vi "03 cDAQ Chan Tester.vi"(7 "Tasks In":refnum<k21>[](array[refnum]), 8 "error in (no error)":errorcluster, 9 "Stream Voltages to File":bool, 10 "DC Voltages Filename":path, 11 "Mode":T1(ring)) -> (0 "error out":errorcluster, 2 "CDAQ Data Out":dbl[](array[numeric]), 5 "Tasks Out":refnum<k21>[](array[refnum]))   [LabVIEW 2012]
uses:
  Hybrid Water Heater/Experiments/Sensor.ctl
  <vilib>/DAQmx/read.llb/DAQmx Read (Analog 2D DBL NChan NSamp).vi
  <vilib>/DAQmx/miscellaneous.llb/DAQmx Fill In Error Info.vi
  Global Test Variables DPT.vi
  <vilib>/Analysis/NI_AALBase.lvlib
  <resource>/objmgr/daqmx.rc
panel:
  in  "I.DC Event":i32=14
  in  "I.AC Event":i32=6
  out "AC Events":cluster{"Mean":dbl, "StdDev":dbl}[](array[cluster])
  out "DC Voltages":cluster{"Mean":dbl, "StdDev":dbl}[](array[cluster])
  in  "Tab Control":enum32{"Graph", "Settings"}(tab)
  out "Voltages":dbl[][](graph)
  out "AvailSampPerAIChan":u32
  out "AvailSampPerTempChan":u32
  in  "TC Max OK Val":dbl=400.0
  in  "TC Min OK Val":dbl=20.0
  in  "StDev Thresh":dbl=0.2
  in  "Timeout":i32=1000
  out "Temps data":dbl[][](array[numeric]) format="%0.2f"
  out "AI Data":dbl[][](array[numeric]) format="%0.2f"
  out "error ai":errorcluster
  in  "Rate_T":dbl=16.0 caption="Rate" format="%0.2f"
  in  "Rate_AI":dbl=16.0
  in  "CDAQ Data":dbl[](array[numeric])
  in  "End":bool
  in  "I.Bar":i32=5
  out "Bar":cluster{"Mean":dbl, "StdDev":dbl}
  in  "I.Gvol":i32=3
  out "G.Vol":cluster{"Mean":dbl, "StdDev":dbl}
  out "Weight":cluster{"Mean":dbl, "StdDev":dbl}
  in  "I.W":i32=1
  in  "I.Tmp":i32=4
  out "Temp":cluster{"Mean":dbl, "StdDev":dbl}
  out "RH":cluster{"Mean":dbl, "StdDev":dbl}
  in  "I.RH":i32=2
  out "G.Pres.":cluster{"Mean":dbl, "StdDev":dbl}
  in  "I.Gas Pressure":i32
  out "Count":dbl
  in  "Panel 4":T2[][](array[typedef])=[[{"Mean"=0.0, " Std"=0.0, "Color Box"=8585007}, {"Mean"=0.0, " Std"=0.0, "Color Box"=8585007}, {"Mean"=0.0, " Std"=0.0, "Color Box"=8585007}, {"Mean"=0.0, " Std"=0.0, "Color Box"=8585007}, {"Mean"=0.0, " Std"=0.0, "Color Box"=8585007}, {"Mean"=0.0, " Std"=0.0, "Color Box"=8585007}], [{"Mean"=0.0, " Std"=0.0, "Color Box"=8585007}, {"Mean"=0.0, " Std"=0.0, "Color Box"=8585007}, {"Mean"=0.0, " Std"=0.0, "Color Box"=8585007}, {"Mean"=0.0, " Std"=0.0, "Color Box"=8585007}, {"Mean"=0.0, " Std"=0.0, "Color Box"=8585007}, {"Mean"=0.0, " Std"=0.0, "Color Box"=8585007}], [{"Mean"=0.0, " Std"=0.0, "Color Box"=8585007}, {"Mean"=0.0, " Std"=0.0, "Color Box"=8585007}, {"Mean"=0.0, " Std"=0.0, "Color Box"=8585007}, {"Mean"=0.0, " Std"=0.0, "Color Box"=8585007}, {"Mean"=0.0, " Std"=0.0, "Color Box"=8585007}, {"Mean"=0.0, " Std"=0.0, "Color Box"=8585007}]]
  out "Gas Temp":T2={"Mean"=0.0, " Std"=0.0, "Color Box"=8585007}
  in  "Panel 3":T2[][](array[typedef])=[[{"Mean"=0.0, " Std"=0.0, "Color Box"=8585007}, {"Mean"=0.0, " Std"=0.0, "Color Box"=8585007}, {"Mean"=0.0, " Std"=0.0, "Color Box"=8585007}, {"Mean"=0.0, " Std"=0.0, "Color Box"=8585007}, {"Mean"=0.0, " Std"=0.0, "Color Box"=8585007}, {"Mean"=0.0, " Std"=0.0, "Color Box"=8585007}], [{"Mean"=0.0, " Std"=0.0, "Color Box"=8585007}, {"Mean"=0.0, " Std"=0.0, "Color Box"=8585007}, {"Mean"=0.0, " Std"=0.0, "Color Box"=8585007}, {"Mean"=0.0, " Std"=0.0, "Color Box"=8585007}, {"Mean"=0.0, " Std"=0.0, "Color Box"=8585007}, {"Mean"=0.0, " Std"=0.0, "Color Box"=8585007}], [{"Mean"=0.0, " Std"=0.0, "Color Box"=8585007}, {"Mean"=0.0, " Std"=0.0, "Color Box"=8585007}, {"Mean"=0.0, " Std"=0.0, "Color Box"=8585007}, {"Mean"=0.0, " Std"=0.0, "Color Box"=8585007}, {"Mean"=0.0, " Std"=0.0, "Color Box"=8585007}, {"Mean"=0.0, " Std"=0.0, "Color Box"=8585007}]]
  in  "Panel 2":T2[][](array[typedef])=[[{"Mean"=0.0, " Std"=0.0, "Color Box"=8585007}, {"Mean"=0.0, " Std"=0.0, "Color Box"=8585007}, {"Mean"=0.0, " Std"=0.0, "Color Box"=8585007}, {"Mean"=0.0, " Std"=0.0, "Color Box"=8585007}, {"Mean"=0.0, " Std"=0.0, "Color Box"=8585007}, {"Mean"=0.0, " Std"=0.0, "Color Box"=8585007}], [{"Mean"=0.0, " Std"=0.0, "Color Box"=8585007}, {"Mean"=0.0, " Std"=0.0, "Color Box"=8585007}, {"Mean"=0.0, " Std"=0.0, "Color Box"=8585007}, {"Mean"=0.0, " Std"=0.0, "Color Box"=8585007}, {"Mean"=0.0, " Std"=0.0, "Color Box"=8585007}, {"Mean"=0.0, " Std"=0.0, "Color Box"=8585007}], [{"Mean"=0.0, " Std"=0.0, "Color Box"=8585007}, {"Mean"=0.0, " Std"=0.0, "Color Box"=8585007}, {"Mean"=0.0, " Std"=0.0, "Color Box"=8585007}, {"Mean"=0.0, " Std"=0.0, "Color Box"=8585007}, {"Mean"=0.0, " Std"=0.0, "Color Box"=8585007}, {"Mean"=0.0, " Std"=0.0, "Color Box"=8585007}]]
  in  "Panel 1":T2[][](array[typedef])=[[{"Mean"=0.0, " Std"=0.0, "Color Box"=8585007}, {"Mean"=0.0, " Std"=0.0, "Color Box"=8585007}, {"Mean"=0.0, " Std"=0.0, "Color Box"=8585007}, {"Mean"=0.0, " Std"=0.0, "Color Box"=8585007}, {"Mean"=0.0, " Std"=0.0, "Color Box"=8585007}, {"Mean"=0.0, " Std"=0.0, "Color Box"=8585007}], [{"Mean"=0.0, " Std"=0.0, "Color Box"=8585007}, {"Mean"=0.0, " Std"=0.0, "Color Box"=8585007}, {"Mean"=0.0, " Std"=0.0, "Color Box"=8585007}, {"Mean"=0.0, " Std"=0.0, "Color Box"=8585007}, {"Mean"=0.0, " Std"=0.0, "Color Box"=8585007}, {"Mean"=0.0, " Std"=0.0, "Color Box"=8585007}], [{"Mean"=0.0, " Std"=0.0, "Color Box"=8585007}, {"Mean"=0.0, " Std"=0.0, "Color Box"=8585007}, {"Mean"=0.0, " Std"=0.0, "Color Box"=8585007}, {"Mean"=0.0, " Std"=0.0, "Color Box"=8585007}, {"Mean"=0.0, " Std"=0.0, "Color Box"=8585007}, {"Mean"=0.0, " Std"=0.0, "Color Box"=8585007}]]
  in  "Num Samples":i32=5
  in  "Test DAQ":bool
  in  "EXIT":bool
  # "DPT Pannel Channel Tester"
  # "Channel \nGas Pressure 0\nWeight 1\nRH 2\nGas Volume 3\nTemp 4\nBaromentric Pressure 5"
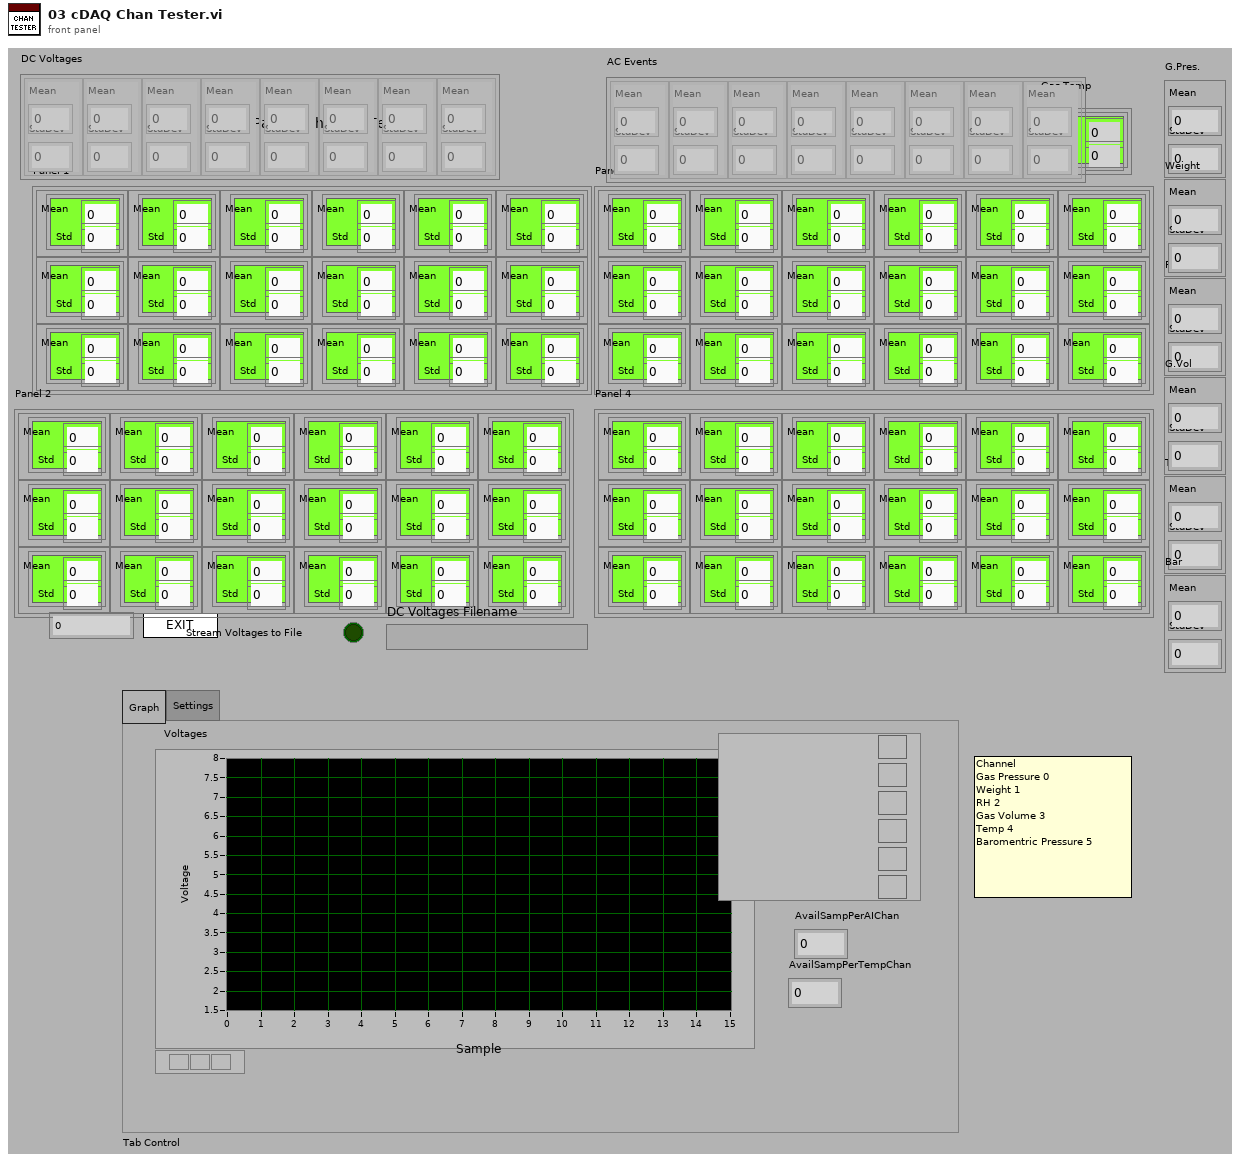
[diagram p1: front panel]
types:
  T1 = enum16{"Exe", "Init CDAQ", "Gather DATA", "Close"}
  T2 = typedef "Sensor.ctl" = cluster{"Mean":dbl, " Std":dbl, "Color Box":u32}
  T3 = enum32{"invalid app kind", "Development System", "Run Time System", "Student Edition", "Embedded LabVIEW", "Evaluation", "Custom"}
  T4 = enum32{"Invalid", "Standard", "Closed", "Hidden", "Minimized", "Maximized"}
  T5 = cluster{"Core":cluster{"Current VI Reference":refnum<vi>, "Close Panel on Exit?":bool}, "Num Samples":i32, "Temp  Data Array":T2[], "AI Data":cluster{"Mean":dbl, "StdDev":dbl}[], "Init":bool, "CDAQ Data":dbl[], "Tasks In":refnum<k21>[], "error in (no error)":errorcluster}
  T6 = cluster{"Current VI Reference":refnum<vi>, "Close Panel on Exit?":bool}
  T7 = typedef "DPT Global Type.ctl" = cluster{"Test Setup":cluster{"RH Resistor":dbl, "Temp Cal":dbl, "Temp Coeff":dbl, "Power On Threshold":dbl, "MA Filter Size":i32, "Weight Offset":dbl, "Temp Resistor":dbl, "Gas Enabled":bool, "Gas P. Resistor":dbl, "Scale Com":dbl, "W. Samps":i32, "Temp4mA Val":dbl, "Temp20mA Val":dbl, "RH4mA Val":dbl, "RH20mA Val":dbl, "GPres4mA Val":dbl, "Gpres20mA Val":dbl, "Smoothing":bool, "CDAQ":bool, "34970":bool, "34980":bool, "RH-IP":string, "RH-IP2":string, "RH-IP3":string, "CompVolume":dbl, "T45_Coeff.":dbl}, "Agilent Setup":cluster{"Scale Channel":string, "TC Channels":string, "VDC Discrete Channels":string, "RH Chan":string, "Temp Chan":string, "Tscale Channel":string, "RDB Channel":string, "Gas Temperature":string, "Gas Pressure":string, "Barometric Pressure":string, "Gas Feedback Chan":string}, "Directories":cluster{"Work File Directory":path, "Save File Directory":path, "Library Directory":path, "Data Backup Directory":path, "Data Backup Dir Fail":path, "Lab Directory":path}, "Test Information":cluster{"Model:":string, "Temperature:":string, "Engineer:":string, "Technician:":string, "Comments:":string, "Lab ID:":string, "TR Number:":string, "Test Number:":string, "Test Station:":string, "Empty Dryer Cold Weight:":dbl, "Serial Number:":string, "Build:":string, "Dryer Type":string, "Humidity":string, "Test Title per TR:":string}, "cDAQ Array Locations":cluster{"Scale Channel":string, "TC Channels":string, "VDC Discrete Channel":string, "RH Chan":string, "Temp Chan":string, "Tscale Channel":string, "RDB Channel":string, "Gas Temperature":string, "Gas Pressure":string, "Barometric Pressure":string, "Gas Feedback Chan":string}}
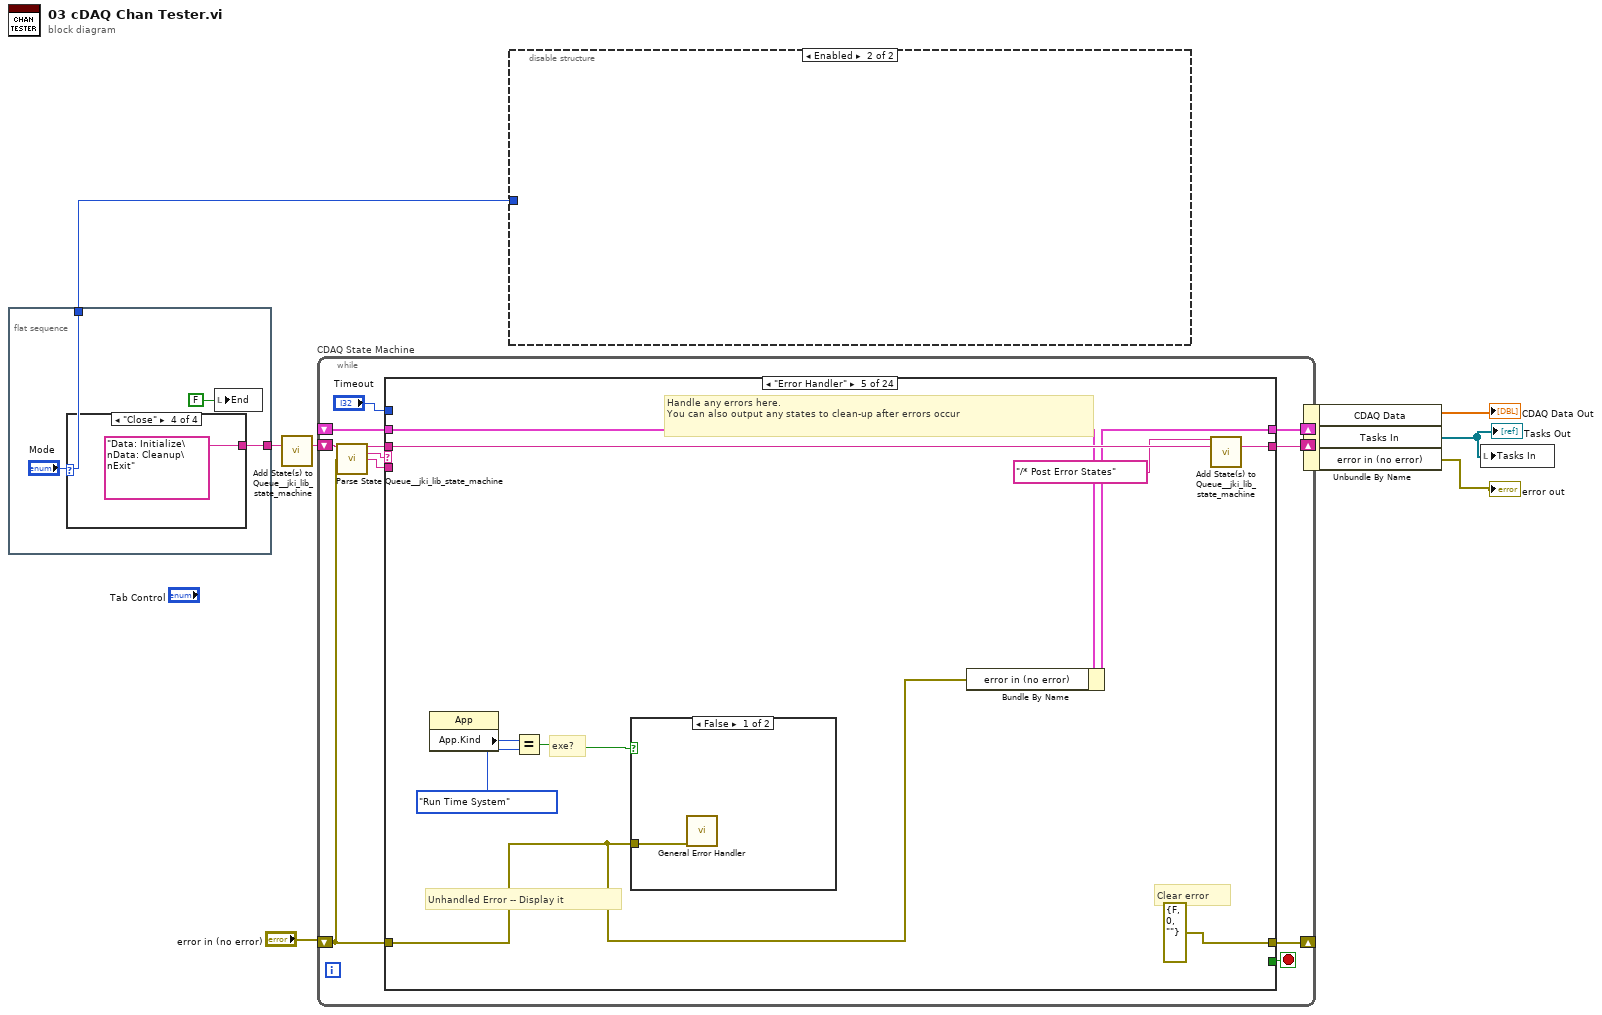
[diagram p0: block diagram]
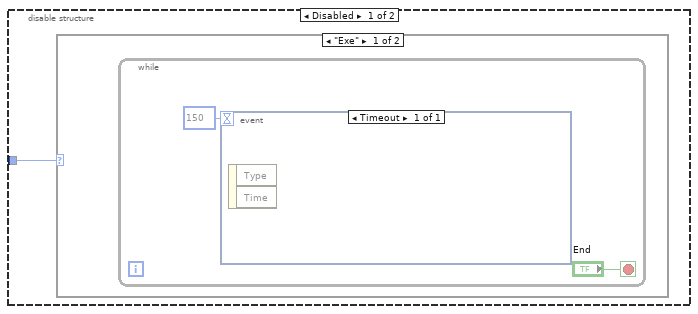
[diagram p2: hidden frame]
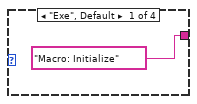
[diagram p4: hidden frame]
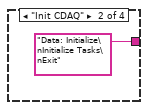
[diagram p5: hidden frame]
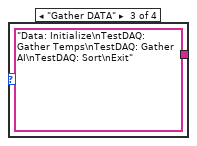
[diagram p6: hidden frame]
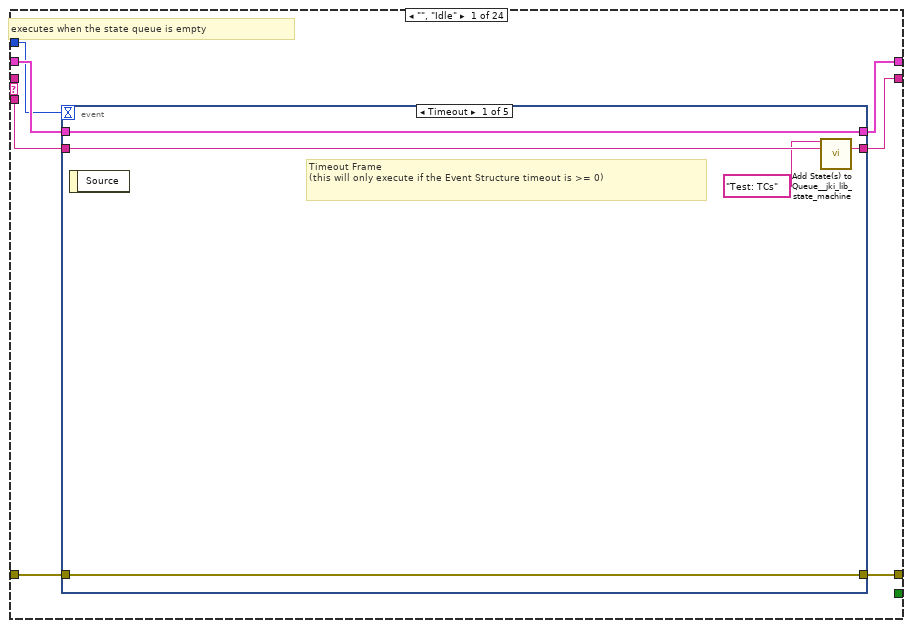
[diagram p7: hidden frame]
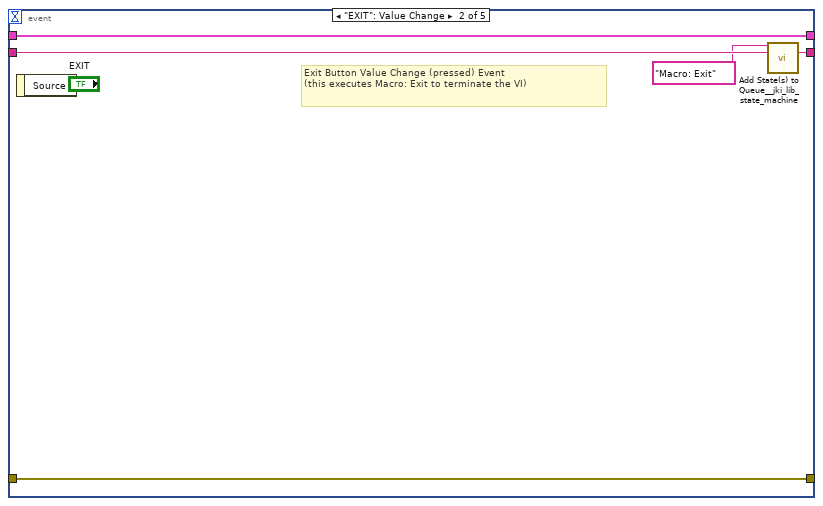
[diagram p8: hidden frame]
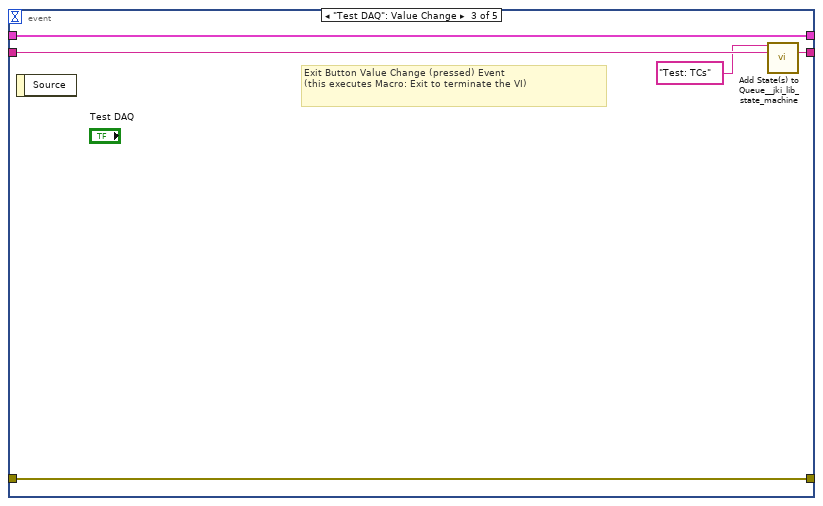
[diagram p9: hidden frame]
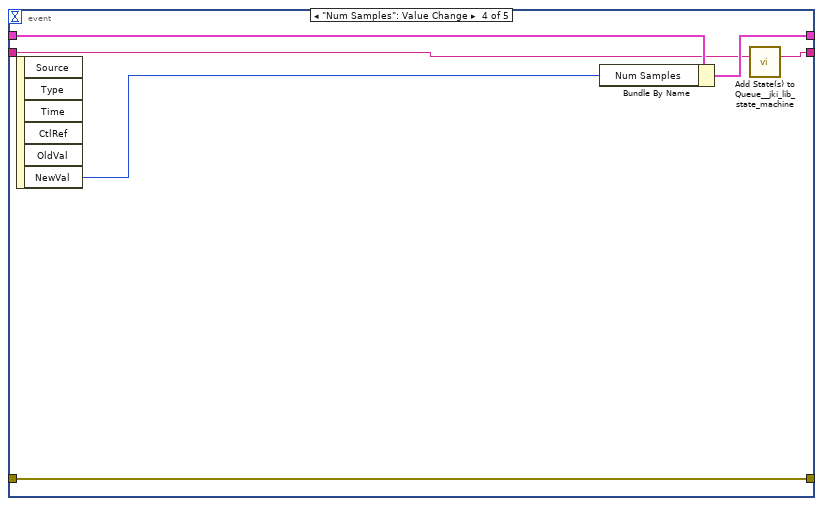
[diagram p10: hidden frame]
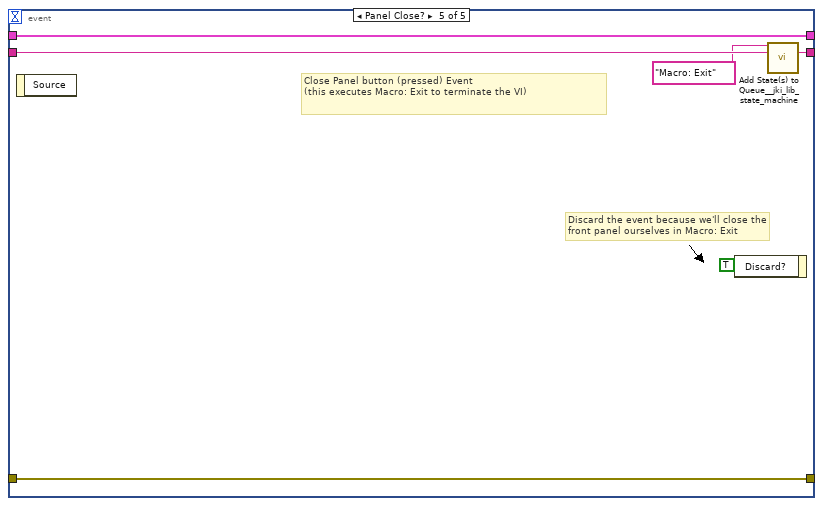
[diagram p11: hidden frame]
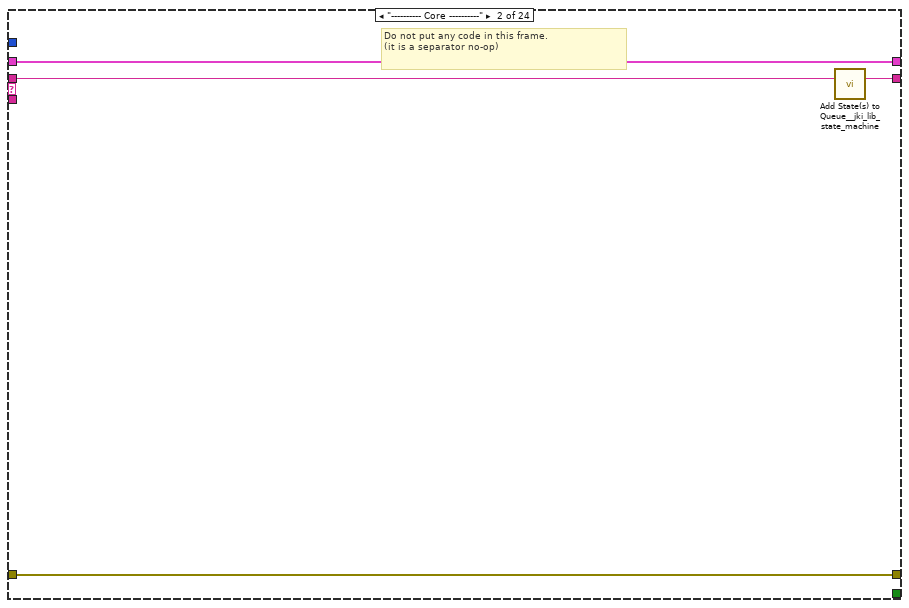
[diagram p12: hidden frame]
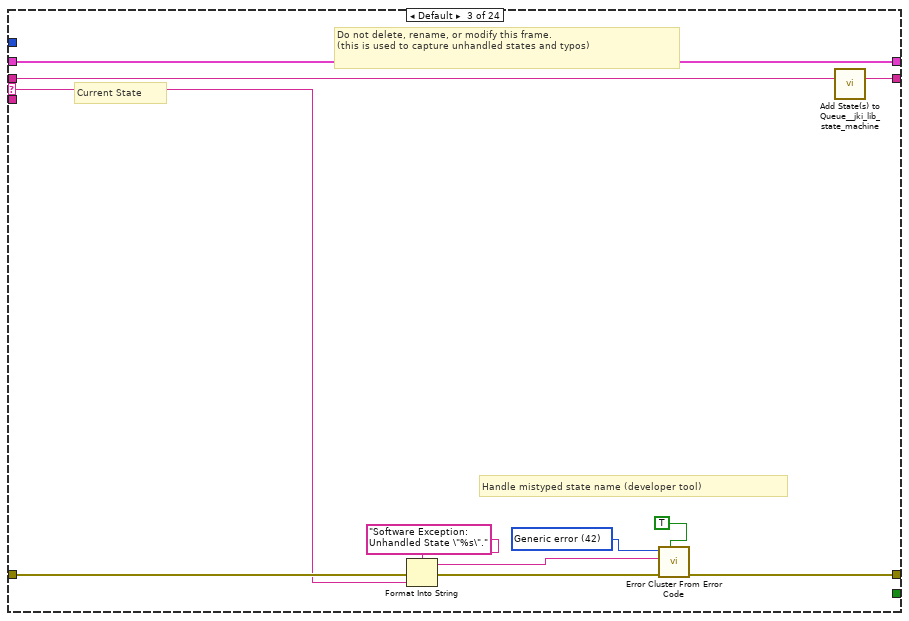
[diagram p13: hidden frame]
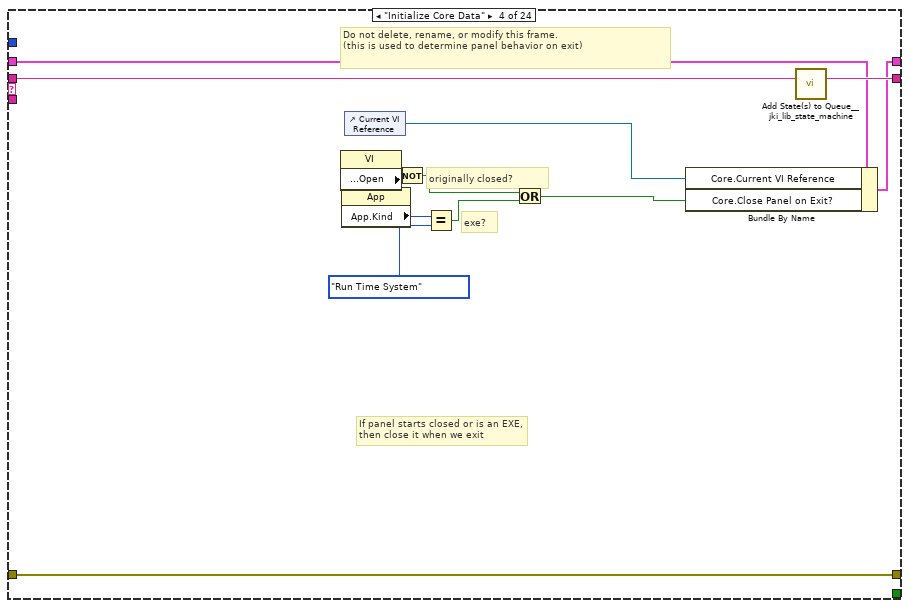
[diagram p14: hidden frame]
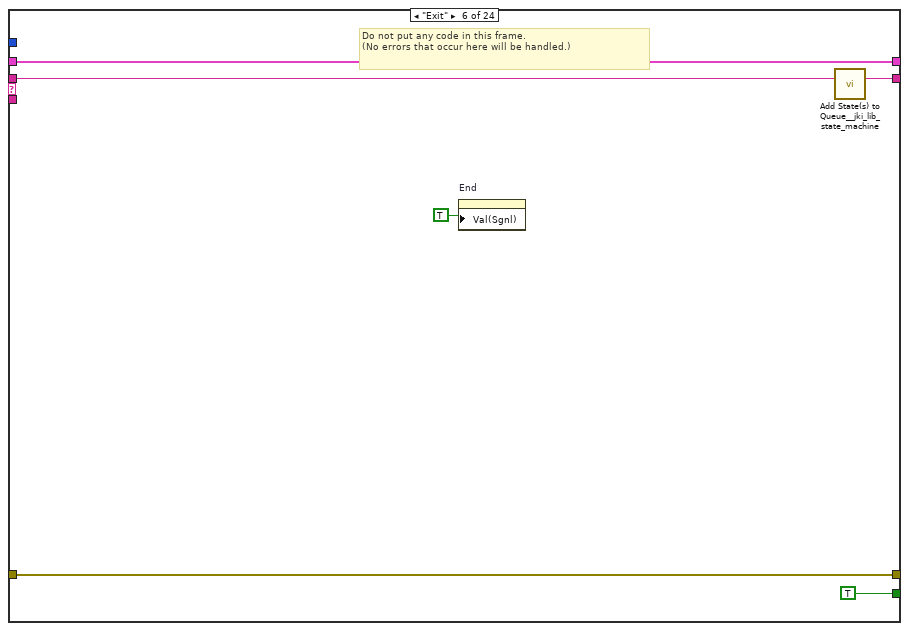
[diagram p16: hidden frame]
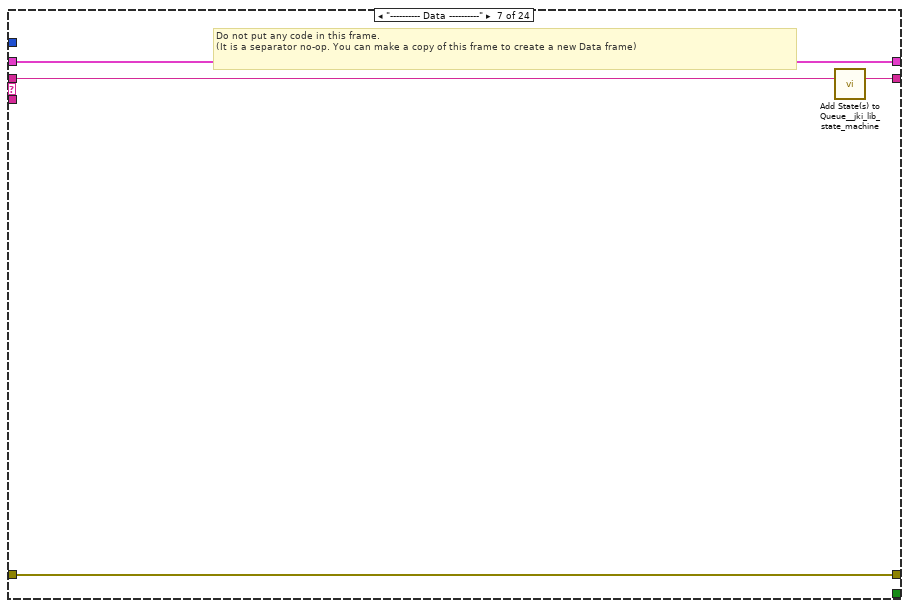
[diagram p17: hidden frame]
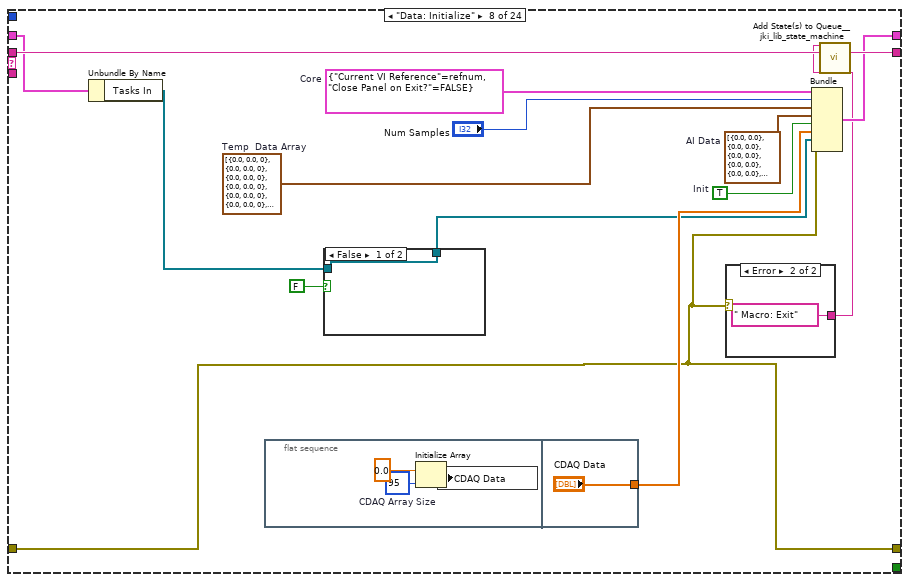
[diagram p18: hidden frame]
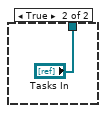
[diagram p19: hidden frame]
diagram:
  n1 = flat-sequence {
    tunnel: [w11] -> w7
    tunnel: ["Mode"] -> w3
    frame #0 {
      n2 = case shown="\"Close\"" "Mode" {
        tunnel: ["Macro: Initialize" "Data: Initialize\nInitialize Tasks\nExit" "Data: Initialize\nTestDAQ: Gather Temps\nTestDAQ: Gather AI\nTestDAQ: Sort\nExit" "Data: Initialize\nData: Cleanup\nExit"] -> w11
        frame "Exe", Default {
        }
        frame "Init CDAQ" {
        }
        frame "Gather DATA" {
        }
        frame "Close" {
        }
      }
      n3 = local write "End"(FALSE ("stop")) -> ()
    }
  }
  n4 = call <vilib>:"Add State(s) to Queue__jki_lib_state_machine.vi"("State(s) in (\"\")"=w7) -> ("States Out"=w8:string)  [unwired: 14 in]
  n5 = while "CDAQ State Machine" {
    shift-right: [w19] -> w5
    shift-left: _ -> [w18]
    shift-right: [w22] -> _
    shift-left: "error in (no error)" -> [w16]
    shift-right: [w21] -> _
    shift-left: w8 -> [w23]
    stop <- w20 stop-if-true
    n6 = call <vilib>:"Parse State Queue__jki_lib_state_machine.vi"("State Queue"=w23, "Error In (no error)"=w16) -> ("Remaining States"=w25:string, "Current State"=w26:string, "Arguments"=w24:string)  [unwired: 11 in]
    n7 = case shown="\"Error Handler\"" w26 {
      selector: w26 -> [_ _ w65 _ _ _ _ _ _ _ _ _ _ _ _ _ _ _ _ _ _ _ _ _]
      tunnel: w25 -> [w33 w64 w69 w87 w97 w104 w108 w123 w145 w154 w164 w174 w192 w203 w229 w234 w244 w248 w253 w257 w275 w317 w358 w605]
      tunnel: w24 -> [_ _ _ _ _ _ _ _ _ _ _ _ w187 w197 _ _ _ _ _ _ _ _ _ _]
      tunnel: w18 -> [w31 w61 w67 w78 w94 w102 w105 w113 w139 w151 w161 w172 w190 w199 w226 w231 w241 w245 w251 w254 w273 w315 w352 w602]
      tunnel: [w30 w62 w71 w84 errorcluster {"status"=FALSE, "code"=0, "source"=""} ("error out") w101 w106 w109 w141 w152 w162 w171 w188 w200 w227 w232 w242 w246 w249 w255 w261 w307 w356 w603] -> w22
      tunnel: w16 -> [w29 w62 w70 w84 w88 w101 w106 w109 w143 w150 w162 w171 w189 w201 w227 w232 w242 w246 w249 w255 w260 w312 w356 w603]
      tunnel: [w32 w63 w68 w86 w96 w103 w107 w122 w144 w153 w163 w173 w191 w202 w228 w233 w243 w247 w252 w256 w274 w316 w357 w604] -> w21
      tunnel: [_ _ _ _ _ TRUE _ _ _ _ _ _ _ _ _ _ _ _ _ _ _ _ _ _] -> w20
      tunnel: [w28 w61 w67 w85 w92 w102 w105 w121 w138 w151 w161 w172 w190 w199 w226 w231 w241 w245 w251 w254 w271 w313 w351 w602] -> w19
      tunnel: "Timeout" -> [w27 _ _ _ _ _ _ _ _ _ _ _ _ _ _ _ _ _ _ _ _ _ _ _]
      frame "", "Idle" {
        # "executes when the state queue is empty"
        n8 = event shown="[0] Timeout" {
          selector: _ -> [_ _ _ _ _]
          dyn-events: _ -> [_ _ _ _ _]
          timeout: w27 -> [_ _ _ _ _]
          tunnel: w33 -> [w38 w43 w48 w52 w60]
          tunnel: [w37 w42 w47 w51 w59] -> w32
          tunnel: w31 -> [w35 w40 w45 w54 w57]
          tunnel: [w36 w41 w46 w50 w58] -> w30
          tunnel: w29 -> [w36 w41 w46 w50 w58]
          tunnel: [w35 w40 w45 w53 w57] -> w28
          event Timeout {
            # "Timeout Frame\n(this will only execute if the Event Structure timeout is >= 0)"
            n9 = event-data() -> ()  [unwired: 1 in, 1 out]
            n10 = call <vilib>:"Add State(s) to Queue__jki_lib_state_machine.vi"("State(s) in Front (\"\")"="Test: TCs", "State(s) in (\"\")"=w38) -> ("States Out"=w37:string)  [unwired: 13 in]
          }
          event "EXIT": Value Change {
            # "Exit Button Value Change (pressed) Event\n(this executes Macro: Exit to terminate the VI)"
            n11 = event-data() -> ()  [unwired: 1 in, 1 out]
            n12 = call <vilib>:"Add State(s) to Queue__jki_lib_state_machine.vi"("State(s) in Front (\"\")"="Macro: Exit", "State(s) in (\"\")"=w43) -> ("States Out"=w42:string)  [unwired: 13 in]
          }
          event "Test DAQ": Value Change {
            # "Exit Button Value Change (pressed) Event\n(this executes Macro: Exit to terminate the VI)"
            n13 = event-data() -> ()  [unwired: 1 in, 1 out]
            n14 = call <vilib>:"Add State(s) to Queue__jki_lib_state_machine.vi"("State(s) in Front (\"\")"="Test: TCs", "State(s) in (\"\")"=w48) -> ("States Out"=w47:string)  [unwired: 13 in]
          }
          event "Num Samples": Value Change {
            n15 = event-data() -> ("NewVal"=w49:i32)  [unwired: 1 in, 5 out]
            n16 = Bundle By Name(cluster=w54, "Num Samples"=w49) -> (w53:T5)
            n17 = call <vilib>:"Add State(s) to Queue__jki_lib_state_machine.vi"("State(s) in (\"\")"=w52) -> ("States Out"=w51:string)  [unwired: 14 in]
          }
          event Panel Close? {
            # "Discard the event because we'll close the front panel ourselves in Macro: Exit"
            # "Close Panel button (pressed) Event\n(this executes Macro: Exit to terminate the VI)"
            n18 = event-data() -> ()  [unwired: 1 in, 1 out]
            n19 = event-data("Discard?"=TRUE) -> ()  [unwired: 1 in, 1 out]
            n20 = call <vilib>:"Add State(s) to Queue__jki_lib_state_machine.vi"("State(s) in Front (\"\")"="Macro: Exit", "State(s) in (\"\")"=w60) -> ("States Out"=w59:string)  [unwired: 13 in]
          }
        }
      }
      frame "---------- Core ----------" {
        # "Do not put any code in this frame.\n(it is a separator no-op)"
        n21 = call <vilib>:"Add State(s) to Queue__jki_lib_state_machine.vi"("State(s) in (\"\")"=w64) -> ("States Out"=w63:string)  [unwired: 14 in]
      }
      frame Default {
        w74 = 42 items=["No error", "Argument error", "Memory is full", "Out of zone", "End of file", "File already open", "Generic file I/O error", "File not found", "File permission error", "Disk is full", "Duplicate path", "Too many files open", "System feature not enabled", "Resource file not found", "Cannot add resource", "Resource not found", "Image not found", "Image memory error", "Pen does not exist", "Config type invalid", "Config token not found", "Config parse error", "Config memory error", "Bad external code format", "Bad external code offset", "External code not present", "Null window", "Destroy window error", "Null menu", "Print aborted", "Bad print record", "Print driver error", "Windows error during printing", "Memory error during printing", "Print dialog error", "Generic print error", "Invalid device refnum", "Device not found", "Device parameter error", "Device unit error", "Cannot open device", "Device call aborted", "Generic error", "Cancelled by user", "Object ID too low", "Object ID too high", "Object not in heap", "Unknown heap", "Unknown object (invalid DefProc)", "Unknown object (DefProc not in table)", "Message out of range", "Invalid (null) method", "Unknown message", "Manager call not supported", "Bad address", "Network operation in progress", "Network operation timed out", "Connection is busy", "Network attribute not supported", "Network error", "Address in use", "System out of memory", "Connection aborted", "Connection refused", "Not connected", "Already connected", "Connection closed", "Initialization error (interapplication manager)", "Bad occurrence", "Wait on unbound occurrence handler", "Occurrence queue overflow", "Datalog type conflict", "Unused", "Unrecognized type (interapplication manager)", "Memory corrupt", "Failed to make temporary DLL", "Old CIN version", "Drag socket not found", "Failed to load drop-object", "Failed to register OLE object", "Failed to release OLE object", "Format specifier type mismatch", "Unknown format specifier", "Too few format specifiers", "Too many format specifiers", "Scan failed", "Newer CIN version", "Error converting to variant", "Runtime menu error", "Password tampered", "Variant attribute not found", "Incompatible variant data type", "Event data is not available", "Event Store is not present", "Occurrence is not found", "Event Queue is not created", "Event info is not available", "Refnum passed is NULL", "Error retrieving Class GUID", "Error retrieving CoClass GUID", "Error retrieving TypeLib GUID.", "Bad built application magic bytes.", "Specific driver is different from the specific driver associated with the Logical Name.", "There is no session opened to the class driver.", "Max Error", "MAX - Error with config objects", "MAX - Error loading configuration", "MAX - Group not supported"]
        # "Current State"
        # "Do not delete, rename, or modify this frame.\n(this is used to capture unhandled states and typos)"
        # "Handle mistyped state name (developer tool)"
        n22 = Format Into String(format string="Software Exception: Unhandled State \"%s\"." ("message"), error in=w70, w65) -> (resulting string=w73:string, error out=w72:errorcluster)  [unwired: 1 in]
        n23 = call <vilib>:"Error Cluster From Error Code.vi"("show call chain? (False)"=TRUE, "error in (no error)"=w72, "error message (\"\")"=w73, "error code (0)"=w74) -> ("error out"=w71:errorcluster)  [unwired: 5 in]
        n24 = call <vilib>:"Add State(s) to Queue__jki_lib_state_machine.vi"("State(s) in (\"\")"=w69) -> ("States Out"=w68:string)  [unwired: 14 in]
      }
      frame "Initialize Core Data" {
        # "Do not delete, rename, or modify this frame.\n(this is used to determine panel behavior on exit)"
        # "originally closed?"
        # "exe?"
        # "If panel starts closed or is an EXE, then close it when we exit"
        n25 = property class="VI"() -> ("Front Panel.Open"=w83:bool)  [unwired: 2 in, 2 out]
        n26 = property class="App"() -> ("App.Kind"=w82:T3)  [unwired: 2 in, 2 out]
        n27 = control-ref of="Current VI Reference"() -> (w76:refnum<vi>)
        n28 = Not(x=w83) -> (.not. x?=w80:bool)
        n29 = Equal?(x=w82, y=T3."Run Time System" ("Application:Kind")) -> (x = y?=w79:bool)
        n30 = Or(x=w80, y=w79) -> (x .or. y?=w77:bool)
        n31 = Bundle By Name(cluster=w78, "Core.Current VI Reference"=w76, "Core.Close Panel on Exit?"=w77) -> (w85:T5)
        n32 = call <vilib>:"Add State(s) to Queue__jki_lib_state_machine.vi"("State(s) in (\"\")"=w87) -> ("States Out"=w86:string)  [unwired: 14 in]
      }
      frame "Error Handler" {
        # "exe?"
        # "Unhandled Error -- Display it"
        # "Handle any errors here.\nYou can also output any states to clean-up after errors occur"
        # "Clear error"
        n33 = property class="App"() -> ("App.Kind"=w91:T3)  [unwired: 2 in, 2 out]
        n34 = Equal?(x=w91, y=T3."Run Time System" ("Application:Kind")) -> (x = y?=w89:bool)
        n35 = case shown="False" w89 {
          tunnel: w88 -> [w98 _]
          frame False {
            n36 = call <vilib>:"General Error Handler.vi"("error in (no error)"=w98) -> ()  [unwired: 10 in, 5 out]
          }
          frame True {
          }
        }
        n37 = Bundle By Name(cluster=w94, "error in (no error)"=w88) -> (w92:T5)
        n38 = call <vilib>:"Add State(s) to Queue__jki_lib_state_machine.vi"("State(s) in Front (\"\")"="/* Post Error States", "State(s) in (\"\")"=w97) -> ("States Out"=w96:string)  [unwired: 13 in]
      }
      frame "Exit" {
        # "Do not put any code in this frame.\n(No errors that occur here will be handled.)"
        n39 = property on="End" class="Bool (strict)"("Val(Sgnl)"=TRUE ("Value (Signaling)")) -> ()  [unwired: 2 in, 2 out]
        n40 = call <vilib>:"Add State(s) to Queue__jki_lib_state_machine.vi"("State(s) in (\"\")"=w104) -> ("States Out"=w103:string)  [unwired: 14 in]
      }
      frame "---------- Data ----------" {
        # "Do not put any code in this frame.\n(It is a separator no-op. You can make a copy of this frame to create a new Data frame)"
        n41 = call <vilib>:"Add State(s) to Queue__jki_lib_state_machine.vi"("State(s) in (\"\")"=w108) -> ("States Out"=w107:string)  [unwired: 14 in]
      }
      frame "Data: Initialize" {
        w115 = TRUE  # Init
        w117 = cluster{"Mean":dbl, "StdDev":dbl}[] [{"Mean"=0.0, "StdDev"=0.0}, {"Mean"=0.0, "StdDev"=0.0}, {"Mean"=0.0, "StdDev"=0.0}, {"Mean"=0.0, "StdDev"=0.0}, {"Mean"=0.0, "StdDev"=0.0}, {"Mean"=0.0, "StdDev"=0.0}, {"Mean"=0.0, "StdDev"=0.0}, {"Mean"=0.0, "StdDev"=0.0}, {"Mean"=0.0, "StdDev"=0.0}, {"Mean"=0.0, "StdDev"=0.0}, {"Mean"=0.0, "StdDev"=0.0}, {"Mean"=0.0, "StdDev"=0.0}, {"Mean"=0.0, "StdDev"=0.0}, {"Mean"=0.0, "StdDev"=0.0}, {"Mean"=0.0, "StdDev"=0.0}, {"Mean"=0.0, "StdDev"=0.0}]  # AI Data
        w118 = T2[] [{"Mean"=0.0, " Std"=0.0, "Color Box"=0}, {"Mean"=0.0, " Std"=0.0, "Color Box"=0}, {"Mean"=0.0, " Std"=0.0, "Color Box"=0}, {"Mean"=0.0, " Std"=0.0, "Color Box"=0}, {"Mean"=0.0, " Std"=0.0, "Color Box"=0}, {"Mean"=0.0, " Std"=0.0, "Color Box"=0}, {"Mean"=0.0, " Std"=0.0, "Color Box"=0}, {"Mean"=0.0, " Std"=0.0, "Color Box"=0}, {"Mean"=0.0, " Std"=0.0, "Color Box"=0}, {"Mean"=0.0, " Std"=0.0, "Color Box"=0}, {"Mean"=0.0, " Std"=0.0, "Color Box"=0}, {"Mean"=0.0, " Std"=0.0, "Color Box"=0}, {"Mean"=0.0, " Std"=0.0, "Color Box"=0}, {"Mean"=0.0, " Std"=0.0, "Color Box"=0}, {"Mean"=0.0, " Std"=0.0, "Color Box"=0}, {"Mean"=0.0, " Std"=0.0, "Color Box"=0}, {"Mean"=0.0, " Std"=0.0, "Color Box"=0}, {"Mean"=0.0, " Std"=0.0, "Color Box"=0}, {"Mean"=0.0, " Std"=0.0, "Color Box"=0}, {"Mean"=0.0, " Std"=0.0, "Color Box"=0}, {"Mean"=0.0, " Std"=0.0, "Color Box"=0}, {"Mean"=0.0, " Std"=0.0, "Color Box"=0}, {"Mean"=0.0, " Std"=0.0, "Color Box"=0}, {"Mean"=0.0, " Std"=0.0, "Color Box"=0}, {"Mean"=0.0, " Std"=0.0, "Color Box"=0}, {"Mean"=0.0, " Std"=0.0, "Color Box"=0}, {"Mean"=0.0, " Std"=0.0, "Color Box"=0}, {"Mean"=0.0, " Std"=0.0, "Color Box"=0}, {"Mean"=0.0, " Std"=0.0, "Color Box"=0}, {"Mean"=0.0, " Std"=0.0, "Color Box"=0}, {"Mean"=0.0, " Std"=0.0, "Color Box"=0}, {"Mean"=0.0, " Std"=0.0, "Color Box"=0}, {"Mean"=0.0, " Std"=0.0, "Color Box"=0}, {"Mean"=0.0, " Std"=0.0, "Color Box"=0}, {"Mean"=0.0, " Std"=0.0, "Color Box"=0}, {"Mean"=0.0, " Std"=0.0, "Color Box"=0}, {"Mean"=0.0, " Std"=0.0, "Color Box"=0}, {"Mean"=0.0, " Std"=0.0, "Color Box"=0}, {"Mean"=0.0, " Std"=0.0, "Color Box"=0}, {"Mean"=0.0, " Std"=0.0, "Color Box"=0}, {"Mean"=0.0, " Std"=0.0, "Color Box"=0}, {"Mean"=0.0, " Std"=0.0, "Color Box"=0}, {"Mean"=0.0, " Std"=0.0, "Color Box"=0}, {"Mean"=0.0, " Std"=0.0, "Color Box"=0}, {"Mean"=0.0, " Std"=0.0, "Color Box"=0}, {"Mean"=0.0, " Std"=0.0, "Color Box"=0}, {"Mean"=0.0, " Std"=0.0, "Color Box"=0}, {"Mean"=0.0, " Std"=0.0, "Color Box"=0}, {"Mean"=0.0, " Std"=0.0, "Color Box"=0}, {"Mean"=0.0, " Std"=0.0, "Color Box"=0}, {"Mean"=0.0, " Std"=0.0, "Color Box"=0}, {"Mean"=0.0, " Std"=0.0, "Color Box"=0}, {"Mean"=0.0, " Std"=0.0, "Color Box"=0}, {"Mean"=0.0, " Std"=0.0, "Color Box"=0}, {"Mean"=0.0, " Std"=0.0, "Color Box"=0}, {"Mean"=0.0, " Std"=0.0, "Color Box"=0}, {"Mean"=0.0, " Std"=0.0, "Color Box"=0}, {"Mean"=0.0, " Std"=0.0, "Color Box"=0}, {"Mean"=0.0, " Std"=0.0, "Color Box"=0}, {"Mean"=0.0, " Std"=0.0, "Color Box"=0}, {"Mean"=0.0, " Std"=0.0, "Color Box"=0}, {"Mean"=0.0, " Std"=0.0, "Color Box"=0}, {"Mean"=0.0, " Std"=0.0, "Color Box"=0}, {"Mean"=0.0, " Std"=0.0, "Color Box"=0}, {"Mean"=0.0, " Std"=0.0, "Color Box"=0}, {"Mean"=0.0, " Std"=0.0, "Color Box"=0}, {"Mean"=0.0, " Std"=0.0, "Color Box"=0}, {"Mean"=0.0, " Std"=0.0, "Color Box"=0}, {"Mean"=0.0, " Std"=0.0, "Color Box"=0}, {"Mean"=0.0, " Std"=0.0, "Color Box"=0}, {"Mean"=0.0, " Std"=0.0, "Color Box"=0}, {"Mean"=0.0, " Std"=0.0, "Color Box"=0}, {"Mean"=0.0, " Std"=0.0, "Color Box"=0}, {"Mean"=0.0, " Std"=0.0, "Color Box"=0}, {"Mean"=0.0, " Std"=0.0, "Color Box"=0}, {"Mean"=0.0, " Std"=0.0, "Color Box"=0}, {"Mean"=0.0, " Std"=0.0, "Color Box"=0}, {"Mean"=0.0, " Std"=0.0, "Color Box"=0}, {"Mean"=0.0, " Std"=0.0, "Color Box"=0}, {"Mean"=0.0, " Std"=0.0, "Color Box"=0}, {"Mean"=0.0, " Std"=0.0, "Color Box"=0}, {"Mean"=0.0, " Std"=0.0, "Color Box"=0}, {"Mean"=0.0, " Std"=0.0, "Color Box"=0}, {"Mean"=0.0, " Std"=0.0, "Color Box"=0}, {"Mean"=0.0, " Std"=0.0, "Color Box"=0}, {"Mean"=0.0, " Std"=0.0, "Color Box"=0}, {"Mean"=0.0, " Std"=0.0, "Color Box"=0}, {"Mean"=0.0, " Std"=0.0, "Color Box"=0}, {"Mean"=0.0, " Std"=0.0, "Color Box"=0}, {"Mean"=0.0, " Std"=0.0, "Color Box"=0}, {"Mean"=0.0, " Std"=0.0, "Color Box"=0}, {"Mean"=0.0, " Std"=0.0, "Color Box"=0}, {"Mean"=0.0, " Std"=0.0, "Color Box"=0}, {"Mean"=0.0, " Std"=0.0, "Color Box"=0}, {"Mean"=0.0, " Std"=0.0, "Color Box"=0}, {"Mean"=0.0, " Std"=0.0, "Color Box"=0}, {"Mean"=0.0, " Std"=0.0, "Color Box"=0}, {"Mean"=0.0, " Std"=0.0, "Color Box"=0}, {"Mean"=0.0, " Std"=0.0, "Color Box"=0}, {"Mean"=0.0, " Std"=0.0, "Color Box"=0}, {"Mean"=0.0, " Std"=0.0, "Color Box"=0}, {"Mean"=0.0, " Std"=0.0, "Color Box"=0}, {"Mean"=0.0, " Std"=0.0, "Color Box"=0}, {"Mean"=0.0, " Std"=0.0, "Color Box"=0}, {"Mean"=0.0, " Std"=0.0, "Color Box"=0}, {"Mean"=0.0, " Std"=0.0, "Color Box"=0}, {"Mean"=0.0, " Std"=0.0, "Color Box"=0}, {"Mean"=0.0, " Std"=0.0, "Color Box"=0}, {"Mean"=0.0, " Std"=0.0, "Color Box"=0}, {"Mean"=0.0, " Std"=0.0, "Color Box"=0}, {"Mean"=0.0, " Std"=0.0, "Color Box"=0}, {"Mean"=0.0, " Std"=0.0, "Color Box"=0}, {"Mean"=0.0, " Std"=0.0, "Color Box"=0}, {"Mean"=0.0, " Std"=0.0, "Color Box"=0}, {"Mean"=0.0, " Std"=0.0, "Color Box"=0}, {"Mean"=0.0, " Std"=0.0, "Color Box"=0}, {"Mean"=0.0, " Std"=0.0, "Color Box"=0}, {"Mean"=0.0, " Std"=0.0, "Color Box"=0}, {"Mean"=0.0, " Std"=0.0, "Color Box"=0}, {"Mean"=0.0, " Std"=0.0, "Color Box"=0}, {"Mean"=0.0, " Std"=0.0, "Color Box"=0}, {"Mean"=0.0, " Std"=0.0, "Color Box"=0}, {"Mean"=0.0, " Std"=0.0, "Color Box"=0}, {"Mean"=0.0, " Std"=0.0, "Color Box"=0}, {"Mean"=0.0, " Std"=0.0, "Color Box"=0}, {"Mean"=0.0, " Std"=0.0, "Color Box"=0}, {"Mean"=0.0, " Std"=0.0, "Color Box"=0}, {"Mean"=0.0, " Std"=0.0, "Color Box"=0}, {"Mean"=0.0, " Std"=0.0, "Color Box"=0}, {"Mean"=0.0, " Std"=0.0, "Color Box"=0}, {"Mean"=0.0, " Std"=0.0, "Color Box"=0}, {"Mean"=0.0, " Std"=0.0, "Color Box"=0}, {"Mean"=0.0, " Std"=0.0, "Color Box"=0}, {"Mean"=0.0, " Std"=0.0, "Color Box"=0}, {"Mean"=0.0, " Std"=0.0, "Color Box"=0}, {"Mean"=0.0, " Std"=0.0, "Color Box"=0}, {"Mean"=0.0, " Std"=0.0, "Color Box"=0}, {"Mean"=0.0, " Std"=0.0, "Color Box"=0}, {"Mean"=0.0, " Std"=0.0, "Color Box"=0}, {"Mean"=0.0, " Std"=0.0, "Color Box"=0}, {"Mean"=0.0, " Std"=0.0, "Color Box"=0}, {"Mean"=0.0, " Std"=0.0, "Color Box"=0}, {"Mean"=0.0, " Std"=0.0, "Color Box"=0}, {"Mean"=0.0, " Std"=0.0, "Color Box"=0}, {"Mean"=0.0, " Std"=0.0, "Color Box"=0}, {"Mean"=0.0, " Std"=0.0, "Color Box"=0}, {"Mean"=0.0, " Std"=0.0, "Color Box"=0}, {"Mean"=0.0, " Std"=0.0, "Color Box"=0}, {"Mean"=0.0, " Std"=0.0, "Color Box"=0}, {"Mean"=0.0, " Std"=0.0, "Color Box"=0}, {"Mean"=0.0, " Std"=0.0, "Color Box"=0}, {"Mean"=0.0, " Std"=0.0, "Color Box"=0}, {"Mean"=0.0, " Std"=0.0, "Color Box"=0}, {"Mean"=0.0, " Std"=0.0, "Color Box"=0}, {"Mean"=0.0, " Std"=0.0, "Color Box"=0}, {"Mean"=0.0, " Std"=0.0, "Color Box"=0}, {"Mean"=0.0, " Std"=0.0, "Color Box"=0}, {"Mean"=0.0, " Std"=0.0, "Color Box"=0}, {"Mean"=0.0, " Std"=0.0, "Color Box"=0}, {"Mean"=0.0, " Std"=0.0, "Color Box"=0}, {"Mean"=0.0, " Std"=0.0, "Color Box"=0}, {"Mean"=0.0, " Std"=0.0, "Color Box"=0}, {"Mean"=0.0, " Std"=0.0, "Color Box"=0}, {"Mean"=0.0, " Std"=0.0, "Color Box"=0}, {"Mean"=0.0, " Std"=0.0, "Color Box"=0}, {"Mean"=0.0, " Std"=0.0, "Color Box"=0}, {"Mean"=0.0, " Std"=0.0, "Color Box"=0}, {"Mean"=0.0, " Std"=0.0, "Color Box"=0}, {"Mean"=0.0, " Std"=0.0, "Color Box"=0}, {"Mean"=0.0, " Std"=0.0, "Color Box"=0}, {"Mean"=0.0, " Std"=0.0, "Color Box"=0}, {"Mean"=0.0, " Std"=0.0, "Color Box"=0}, {"Mean"=0.0, " Std"=0.0, "Color Box"=0}, {"Mean"=0.0, " Std"=0.0, "Color Box"=0}, {"Mean"=0.0, " Std"=0.0, "Color Box"=0}, {"Mean"=0.0, " Std"=0.0, "Color Box"=0}, {"Mean"=0.0, " Std"=0.0, "Color Box"=0}, {"Mean"=0.0, " Std"=0.0, "Color Box"=0}, {"Mean"=0.0, " Std"=0.0, "Color Box"=0}, {"Mean"=0.0, " Std"=0.0, "Color Box"=0}, {"Mean"=0.0, " Std"=0.0, "Color Box"=0}, {"Mean"=0.0, " Std"=0.0, "Color Box"=0}, {"Mean"=0.0, " Std"=0.0, "Color Box"=0}, {"Mean"=0.0, " Std"=0.0, "Color Box"=0}, {"Mean"=0.0, " Std"=0.0, "Color Box"=0}, {"Mean"=0.0, " Std"=0.0, "Color Box"=0}, {"Mean"=0.0, " Std"=0.0, "Color Box"=0}, {"Mean"=0.0, " Std"=0.0, "Color Box"=0}, {"Mean"=0.0, " Std"=0.0, "Color Box"=0}, {"Mean"=0.0, " Std"=0.0, "Color Box"=0}, {"Mean"=0.0, " Std"=0.0, "Color Box"=0}, {"Mean"=0.0, " Std"=0.0, "Color Box"=0}, {"Mean"=0.0, " Std"=0.0, "Color Box"=0}, {"Mean"=0.0, " Std"=0.0, "Color Box"=0}, {"Mean"=0.0, " Std"=0.0, "Color Box"=0}, {"Mean"=0.0, " Std"=0.0, "Color Box"=0}, {"Mean"=0.0, " Std"=0.0, "Color Box"=0}, {"Mean"=0.0, " Std"=0.0, "Color Box"=0}, {"Mean"=0.0, " Std"=0.0, "Color Box"=0}, {"Mean"=0.0, " Std"=0.0, "Color Box"=0}, {"Mean"=0.0, " Std"=0.0, "Color Box"=0}, {"Mean"=0.0, " Std"=0.0, "Color Box"=0}, {"Mean"=0.0, " Std"=0.0, "Color Box"=0}, {"Mean"=0.0, " Std"=0.0, "Color Box"=0}, {"Mean"=0.0, " Std"=0.0, "Color Box"=0}, {"Mean"=0.0, " Std"=0.0, "Color Box"=0}, {"Mean"=0.0, " Std"=0.0, "Color Box"=0}, {"Mean"=0.0, " Std"=0.0, "Color Box"=0}, {"Mean"=0.0, " Std"=0.0, "Color Box"=0}, {"Mean"=0.0, " Std"=0.0, "Color Box"=0}, {"Mean"=0.0, " Std"=0.0, "Color Box"=0}, {"Mean"=0.0, " Std"=0.0, "Color Box"=0}, {"Mean"=0.0, " Std"=0.0, "Color Box"=0}, {"Mean"=0.0, " Std"=0.0, "Color Box"=0}, {"Mean"=0.0, " Std"=0.0, "Color Box"=0}, {"Mean"=0.0, " Std"=0.0, "Color Box"=0}, {"Mean"=0.0, " Std"=0.0, "Color Box"=0}, {"Mean"=0.0, " Std"=0.0, "Color Box"=0}, {"Mean"=0.0, " Std"=0.0, "Color Box"=0}, {"Mean"=0.0, " Std"=0.0, "Color Box"=0}, {"Mean"=0.0, " Std"=0.0, "Color Box"=0}, {"Mean"=0.0, " Std"=0.0, "Color Box"=0}, {"Mean"=0.0, " Std"=0.0, "Color Box"=0}, {"Mean"=0.0, " Std"=0.0, "Color Box"=0}, {"Mean"=0.0, " Std"=0.0, "Color Box"=0}, {"Mean"=0.0, " Std"=0.0, "Color Box"=0}, {"Mean"=0.0, " Std"=0.0, "Color Box"=0}, {"Mean"=0.0, " Std"=0.0, "Color Box"=0}, {"Mean"=0.0, " Std"=0.0, "Color Box"=0}, {"Mean"=0.0, " Std"=0.0, "Color Box"=0}, {"Mean"=0.0, " Std"=0.0, "Color Box"=0}, {"Mean"=0.0, " Std"=0.0, "Color Box"=0}, {"Mean"=0.0, " Std"=0.0, "Color Box"=0}, {"Mean"=0.0, " Std"=0.0, "Color Box"=0}, {"Mean"=0.0, " Std"=0.0, "Color Box"=0}, {"Mean"=0.0, " Std"=0.0, "Color Box"=0}, {"Mean"=0.0, " Std"=0.0, "Color Box"=0}, {"Mean"=0.0, " Std"=0.0, "Color Box"=0}, {"Mean"=0.0, " Std"=0.0, "Color Box"=0}, {"Mean"=0.0, " Std"=0.0, "Color Box"=0}, {"Mean"=0.0, " Std"=0.0, "Color Box"=0}, {"Mean"=0.0, " Std"=0.0, "Color Box"=0}, {"Mean"=0.0, " Std"=0.0, "Color Box"=0}, {"Mean"=0.0, " Std"=0.0, "Color Box"=0}, {"Mean"=0.0, " Std"=0.0, "Color Box"=0}, {"Mean"=0.0, " Std"=0.0, "Color Box"=0}, {"Mean"=0.0, " Std"=0.0, "Color Box"=0}, {"Mean"=0.0, " Std"=0.0, "Color Box"=0}, {"Mean"=0.0, " Std"=0.0, "Color Box"=0}, {"Mean"=0.0, " Std"=0.0, "Color Box"=0}, {"Mean"=0.0, " Std"=0.0, "Color Box"=0}, {"Mean"=0.0, " Std"=0.0, "Color Box"=0}, {"Mean"=0.0, " Std"=0.0, "Color Box"=0}, {"Mean"=0.0, " Std"=0.0, "Color Box"=0}, {"Mean"=0.0, " Std"=0.0, "Color Box"=0}, {"Mean"=0.0, " Std"=0.0, "Color Box"=0}, {"Mean"=0.0, " Std"=0.0, "Color Box"=0}, {"Mean"=0.0, " Std"=0.0, "Color Box"=0}, {"Mean"=0.0, " Std"=0.0, "Color Box"=0}, {"Mean"=0.0, " Std"=0.0, "Color Box"=0}, {"Mean"=0.0, " Std"=0.0, "Color Box"=0}, {"Mean"=0.0, " Std"=0.0, "Color Box"=0}, {"Mean"=0.0, " Std"=0.0, "Color Box"=0}, {"Mean"=0.0, " Std"=0.0, "Color Box"=0}, {"Mean"=0.0, " Std"=0.0, "Color Box"=0}, {"Mean"=0.0, " Std"=0.0, "Color Box"=0}, {"Mean"=0.0, " Std"=0.0, "Color Box"=0}, {"Mean"=0.0, " Std"=0.0, "Color Box"=0}, {"Mean"=0.0, " Std"=0.0, "Color Box"=0}, {"Mean"=0.0, " Std"=0.0, "Color Box"=0}, {"Mean"=0.0, " Std"=0.0, "Color Box"=0}, {"Mean"=0.0, " Std"=0.0, "Color Box"=0}, {"Mean"=0.0, " Std"=0.0, "Color Box"=0}, {"Mean"=0.0, " Std"=0.0, "Color Box"=0}, {"Mean"=0.0, " Std"=0.0, "Color Box"=0}, {"Mean"=0.0, " Std"=0.0, "Color Box"=0}, {"Mean"=0.0, " Std"=0.0, "Color Box"=0}, {"Mean"=0.0, " Std"=0.0, "Color Box"=0}, {"Mean"=0.0, " Std"=0.0, "Color Box"=0}, {"Mean"=0.0, " Std"=0.0, "Color Box"=0}, {"Mean"=0.0, " Std"=0.0, "Color Box"=0}, {"Mean"=0.0, " Std"=0.0, "Color Box"=0}, {"Mean"=0.0, " Std"=0.0, "Color Box"=0}, {"Mean"=0.0, " Std"=0.0, "Color Box"=0}, {"Mean"=0.0, " Std"=0.0, "Color Box"=0}, {"Mean"=0.0, " Std"=0.0, "Color Box"=0}, {"Mean"=0.0, " Std"=0.0, "Color Box"=0}, {"Mean"=0.0, " Std"=0.0, "Color Box"=0}, {"Mean"=0.0, " Std"=0.0, "Color Box"=0}, {"Mean"=0.0, " Std"=0.0, "Color Box"=0}, {"Mean"=0.0, " Std"=0.0, "Color Box"=0}, {"Mean"=0.0, " Std"=0.0, "Color Box"=0}, {"Mean"=0.0, " Std"=0.0, "Color Box"=0}, {"Mean"=0.0, " Std"=0.0, "Color Box"=0}, {"Mean"=0.0, " Std"=0.0, "Color Box"=0}, {"Mean"=0.0, " Std"=0.0, "Color Box"=0}, {"Mean"=0.0, " Std"=0.0, "Color Box"=0}, {"Mean"=0.0, " Std"=0.0, "Color Box"=0}, {"Mean"=0.0, " Std"=0.0, "Color Box"=0}, {"Mean"=0.0, " Std"=0.0, "Color Box"=0}, {"Mean"=0.0, " Std"=0.0, "Color Box"=0}, {"Mean"=0.0, " Std"=0.0, "Color Box"=0}, {"Mean"=0.0, " Std"=0.0, "Color Box"=0}, {"Mean"=0.0, " Std"=0.0, "Color Box"=0}, {"Mean"=0.0, " Std"=0.0, "Color Box"=0}, {"Mean"=0.0, " Std"=0.0, "Color Box"=0}, {"Mean"=0.0, " Std"=0.0, "Color Box"=0}, {"Mean"=0.0, " Std"=0.0, "Color Box"=0}, {"Mean"=0.0, " Std"=0.0, "Color Box"=0}, {"Mean"=0.0, " Std"=0.0, "Color Box"=0}, {"Mean"=0.0, " Std"=0.0, "Color Box"=0}, {"Mean"=0.0, " Std"=0.0, "Color Box"=0}, {"Mean"=0.0, " Std"=0.0, "Color Box"=0}, {"Mean"=0.0, " Std"=0.0, "Color Box"=0}, {"Mean"=0.0, " Std"=0.0, "Color Box"=0}, {"Mean"=0.0, " Std"=0.0, "Color Box"=0}, {"Mean"=0.0, " Std"=0.0, "Color Box"=0}, {"Mean"=0.0, " Std"=0.0, "Color Box"=0}, {"Mean"=0.0, " Std"=0.0, "Color Box"=0}, {"Mean"=0.0, " Std"=0.0, "Color Box"=0}, {"Mean"=0.0, " Std"=0.0, "Color Box"=0}, {"Mean"=0.0, " Std"=0.0, "Color Box"=0}, {"Mean"=0.0, " Std"=0.0, "Color Box"=0}, {"Mean"=0.0, " Std"=0.0, "Color Box"=0}, {"Mean"=0.0, " Std"=0.0, "Color Box"=0}, {"Mean"=0.0, " Std"=0.0, "Color Box"=0}, {"Mean"=0.0, " Std"=0.0, "Color Box"=0}, {"Mean"=0.0, " Std"=0.0, "Color Box"=0}, {"Mean"=0.0, " Std"=0.0, "Color Box"=0}, {"Mean"=0.0, " Std"=0.0, "Color Box"=0}, {"Mean"=0.0, " Std"=0.0, "Color Box"=0}, {"Mean"=0.0, " Std"=0.0, "Color Box"=0}, {"Mean"=0.0, " Std"=0.0, "Color Box"=0}, {"Mean"=0.0, " Std"=0.0, "Color Box"=0}, {"Mean"=0.0, " Std"=0.0, "Color Box"=0}, {"Mean"=0.0, " Std"=0.0, "Color Box"=0}, {"Mean"=0.0, " Std"=0.0, "Color Box"=0}, {"Mean"=0.0, " Std"=0.0, "Color Box"=0}, {"Mean"=0.0, " Std"=0.0, "Color Box"=0}, {"Mean"=0.0, " Std"=0.0, "Color Box"=0}, {"Mean"=0.0, " Std"=0.0, "Color Box"=0}, {"Mean"=0.0, " Std"=0.0, "Color Box"=0}, {"Mean"=0.0, " Std"=0.0, "Color Box"=0}, {"Mean"=0.0, " Std"=0.0, "Color Box"=0}, {"Mean"=0.0, " Std"=0.0, "Color Box"=0}, {"Mean"=0.0, " Std"=0.0, "Color Box"=0}, {"Mean"=0.0, " Std"=0.0, "Color Box"=0}, {"Mean"=0.0, " Std"=0.0, "Color Box"=0}, {"Mean"=0.0, " Std"=0.0, "Color Box"=0}, {"Mean"=0.0, " Std"=0.0, "Color Box"=0}, {"Mean"=0.0, " Std"=0.0, "Color Box"=0}, {"Mean"=0.0, " Std"=0.0, "Color Box"=0}, {"Mean"=0.0, " Std"=0.0, "Color Box"=0}, {"Mean"=0.0, " Std"=0.0, "Color Box"=0}, {"Mean"=0.0, " Std"=0.0, "Color Box"=0}, {"Mean"=0.0, " Std"=0.0, "Color Box"=0}, {"Mean"=0.0, " Std"=0.0, "Color Box"=0}, {"Mean"=0.0, " Std"=0.0, "Color Box"=0}, {"Mean"=0.0, " Std"=0.0, "Color Box"=0}, {"Mean"=0.0, " Std"=0.0, "Color Box"=0}, {"Mean"=0.0, " Std"=0.0, "Color Box"=0}, {"Mean"=0.0, " Std"=0.0, "Color Box"=0}, {"Mean"=0.0, " Std"=0.0, "Color Box"=0}, {"Mean"=0.0, " Std"=0.0, "Color Box"=0}, {"Mean"=0.0, " Std"=0.0, "Color Box"=0}, {"Mean"=0.0, " Std"=0.0, "Color Box"=0}, {"Mean"=0.0, " Std"=0.0, "Color Box"=0}, {"Mean"=0.0, " Std"=0.0, "Color Box"=0}, {"Mean"=0.0, " Std"=0.0, "Color Box"=0}, {"Mean"=0.0, " Std"=0.0, "Color Box"=0}, {"Mean"=0.0, " Std"=0.0, "Color Box"=0}, {"Mean"=0.0, " Std"=0.0, "Color Box"=0}, {"Mean"=0.0, " Std"=0.0, "Color Box"=0}, {"Mean"=0.0, " Std"=0.0, "Color Box"=0}, {"Mean"=0.0, " Std"=0.0, "Color Box"=0}, {"Mean"=0.0, " Std"=0.0, "Color Box"=0}, {"Mean"=0.0, " Std"=0.0, "Color Box"=0}, {"Mean"=0.0, " Std"=0.0, "Color Box"=0}, {"Mean"=0.0, " Std"=0.0, "Color Box"=0}, {"Mean"=0.0, " Std"=0.0, "Color Box"=0}, {"Mean"=0.0, " Std"=0.0, "Color Box"=0}, {"Mean"=0.0, " Std"=0.0, "Color Box"=0}, {"Mean"=0.0, " Std"=0.0, "Color Box"=0}, {"Mean"=0.0, " Std"=0.0, "Color Box"=0}, {"Mean"=0.0, " Std"=0.0, "Color Box"=0}, {"Mean"=0.0, " Std"=0.0, "Color Box"=0}, {"Mean"=0.0, " Std"=0.0, "Color Box"=0}, {"Mean"=0.0, " Std"=0.0, "Color Box"=0}, {"Mean"=0.0, " Std"=0.0, "Color Box"=0}, {"Mean"=0.0, " Std"=0.0, "Color Box"=0}, {"Mean"=0.0, " Std"=0.0, "Color Box"=0}, {"Mean"=0.0, " Std"=0.0, "Color Box"=0}, {"Mean"=0.0, " Std"=0.0, "Color Box"=0}, {"Mean"=0.0, " Std"=0.0, "Color Box"=0}, {"Mean"=0.0, " Std"=0.0, "Color Box"=0}, {"Mean"=0.0, " Std"=0.0, "Color Box"=0}, {"Mean"=0.0, " Std"=0.0, "Color Box"=0}, {"Mean"=0.0, " Std"=0.0, "Color Box"=0}, {"Mean"=0.0, " Std"=0.0, "Color Box"=0}, {"Mean"=0.0, " Std"=0.0, "Color Box"=0}, {"Mean"=0.0, " Std"=0.0, "Color Box"=0}, {"Mean"=0.0, " Std"=0.0, "Color Box"=0}, {"Mean"=0.0, " Std"=0.0, "Color Box"=0}, {"Mean"=0.0, " Std"=0.0, "Color Box"=0}, {"Mean"=0.0, " Std"=0.0, "Color Box"=0}, {"Mean"=0.0, " Std"=0.0, "Color Box"=0}, {"Mean"=0.0, " Std"=0.0, "Color Box"=0}, {"Mean"=0.0, " Std"=0.0, "Color Box"=0}, {"Mean"=0.0, " Std"=0.0, "Color Box"=0}, {"Mean"=0.0, " Std"=0.0, "Color Box"=0}, {"Mean"=0.0, " Std"=0.0, "Color Box"=0}, {"Mean"=0.0, " Std"=0.0, "Color Box"=0}, {"Mean"=0.0, " Std"=0.0, "Color Box"=0}, {"Mean"=0.0, " Std"=0.0, "Color Box"=0}, {"Mean"=0.0, " Std"=0.0, "Color Box"=0}, {"Mean"=0.0, " Std"=0.0, "Color Box"=0}, {"Mean"=0.0, " Std"=0.0, "Color Box"=0}, {"Mean"=0.0, " Std"=0.0, "Color Box"=0}, {"Mean"=0.0, " Std"=0.0, "Color Box"=0}, {"Mean"=0.0, " Std"=0.0, "Color Box"=0}, {"Mean"=0.0, " Std"=0.0, "Color Box"=0}, {"Mean"=0.0, " Std"=0.0, "Color Box"=0}, {"Mean"=0.0, " Std"=0.0, "Color Box"=0}, {"Mean"=0.0, " Std"=0.0, "Color Box"=0}, {"Mean"=0.0, " Std"=0.0, "Color Box"=0}, {"Mean"=0.0, " Std"=0.0, "Color Box"=0}, {"Mean"=0.0, " Std"=0.0, "Color Box"=0}, {"Mean"=0.0, " Std"=0.0, "Color Box"=0}, {"Mean"=0.0, " Std"=0.0, "Color Box"=0}, {"Mean"=0.0, " Std"=0.0, "Color Box"=0}, {"Mean"=0.0, " Std"=0.0, "Color Box"=0}, {"Mean"=0.0, " Std"=0.0, "Color Box"=0}, {"Mean"=0.0, " Std"=0.0, "Color Box"=0}, {"Mean"=0.0, " Std"=0.0, "Color Box"=0}, {"Mean"=0.0, " Std"=0.0, "Color Box"=0}, {"Mean"=0.0, " Std"=0.0, "Color Box"=0}, {"Mean"=0.0, " Std"=0.0, "Color Box"=0}, {"Mean"=0.0, " Std"=0.0, "Color Box"=0}, {"Mean"=0.0, " Std"=0.0, "Color Box"=0}, {"Mean"=0.0, " Std"=0.0, "Color Box"=0}, {"Mean"=0.0, " Std"=0.0, "Color Box"=0}, {"Mean"=0.0, " Std"=0.0, "Color Box"=0}, {"Mean"=0.0, " Std"=0.0, "Color Box"=0}, {"Mean"=0.0, " Std"=0.0, "Color Box"=0}, {"Mean"=0.0, " Std"=0.0, "Color Box"=0}, {"Mean"=0.0, " Std"=0.0, "Color Box"=0}, {"Mean"=0.0, " Std"=0.0, "Color Box"=0}, {"Mean"=0.0, " Std"=0.0, "Color Box"=0}, {"Mean"=0.0, " Std"=0.0, "Color Box"=0}, {"Mean"=0.0, " Std"=0.0, "Color Box"=0}, {"Mean"=0.0, " Std"=0.0, "Color Box"=0}, {"Mean"=0.0, " Std"=0.0, "Color Box"=0}, {"Mean"=0.0, " Std"=0.0, "Color Box"=0}, {"Mean"=0.0, " Std"=0.0, "Color Box"=0}, {"Mean"=0.0, " Std"=0.0, "Color Box"=0}, {"Mean"=0.0, " Std"=0.0, "Color Box"=0}, {"Mean"=0.0, " Std"=0.0, "Color Box"=0}, {"Mean"=0.0, " Std"=0.0, "Color Box"=0}, {"Mean"=0.0, " Std"=0.0, "Color Box"=0}, {"Mean"=0.0, " Std"=0.0, "Color Box"=0}, {"Mean"=0.0, " Std"=0.0, "Color Box"=0}, {"Mean"=0.0, " Std"=0.0, "Color Box"=0}, {"Mean"=0.0, " Std"=0.0, "Color Box"=0}, {"Mean"=0.0, " Std"=0.0, "Color Box"=0}, {"Mean"=0.0, " Std"=0.0, "Color Box"=0}, {"Mean"=0.0, " Std"=0.0, "Color Box"=0}, {"Mean"=0.0, " Std"=0.0, "Color Box"=0}, {"Mean"=0.0, " Std"=0.0, "Color Box"=0}, {"Mean"=0.0, " Std"=0.0, "Color Box"=0}, {"Mean"=0.0, " Std"=0.0, "Color Box"=0}, {"Mean"=0.0, " Std"=0.0, "Color Box"=0}, {"Mean"=0.0, " Std"=0.0, "Color Box"=0}, {"Mean"=0.0, " Std"=0.0, "Color Box"=0}, {"Mean"=0.0, " Std"=0.0, "Color Box"=0}, {"Mean"=0.0, " Std"=0.0, "Color Box"=0}, {"Mean"=0.0, " Std"=0.0, "Color Box"=0}, {"Mean"=0.0, " Std"=0.0, "Color Box"=0}, {"Mean"=0.0, " Std"=0.0, "Color Box"=0}, {"Mean"=0.0, " Std"=0.0, "Color Box"=0}, {"Mean"=0.0, " Std"=0.0, "Color Box"=0}, {"Mean"=0.0, " Std"=0.0, "Color Box"=0}, {"Mean"=0.0, " Std"=0.0, "Color Box"=0}, {"Mean"=0.0, " Std"=0.0, "Color Box"=0}, {"Mean"=0.0, " Std"=0.0, "Color Box"=0}, {"Mean"=0.0, " Std"=0.0, "Color Box"=0}, {"Mean"=0.0, " Std"=0.0, "Color Box"=0}, {"Mean"=0.0, " Std"=0.0, "Color Box"=0}, {"Mean"=0.0, " Std"=0.0, "Color Box"=0}, {"Mean"=0.0, " Std"=0.0, "Color Box"=0}, {"Mean"=0.0, " Std"=0.0, "Color Box"=0}, {"Mean"=0.0, " Std"=0.0, "Color Box"=0}, {"Mean"=0.0, " Std"=0.0, "Color Box"=0}, {"Mean"=0.0, " Std"=0.0, "Color Box"=0}, {"Mean"=0.0, " Std"=0.0, "Color Box"=0}, {"Mean"=0.0, " Std"=0.0, "Color Box"=0}, {"Mean"=0.0, " Std"=0.0, "Color Box"=0}, {"Mean"=0.0, " Std"=0.0, "Color Box"=0}, {"Mean"=0.0, " Std"=0.0, "Color Box"=0}, {"Mean"=0.0, " Std"=0.0, "Color Box"=0}, {"Mean"=0.0, " Std"=0.0, "Color Box"=0}, {"Mean"=0.0, " Std"=0.0, "Color Box"=0}]  # Temp  Data Array
        w120 = T6 {"Current VI Reference"=refnum, "Close Panel on Exit?"=FALSE}  # Core
        n42 = Unbundle By Name(w113) -> ("Tasks In"=w110:refnum<k21>[])
        n43 = flat-sequence {
          tunnel: ["CDAQ Data"] -> w114
          frame #0 {
            w127 = 95  # CDAQ Array Size
            n44 = Initialize Array(0.0 ("Mean"), w127) -> (w126:dbl[])
            n45 = local write "CDAQ Data"(w126) -> ()
          }
          frame #1 {
          }
        }
        n46 = case shown="False" FALSE {
          tunnel: [w124 "Tasks In"] -> w112
          tunnel: w110 -> [w124 _]
          frame False {
          }
          frame True {
          }
        }
        n47 = case shown="Error" w109 {
          tunnel: [_ " Macro: Exit" ("State(s) in Front (\"\")")] -> w116
          frame No Error {
          }
          frame Error {
          }
        }
        n48 = Bundle("Core"=w120, "Num Samples"="Num Samples", "Temp  Data Array"=w118, "AI Data"=w117, "Init"=w115, "CDAQ Data"=w114, "Tasks In"=w112, "error in (no error)"=w109) -> (w121:T5)  [unwired: 1 in]
        n49 = call <vilib>:"Add State(s) to Queue__jki_lib_state_machine.vi"("State(s) in Front (\"\")"=w116, "State(s) in (\"\")"=w123) -> ("States Out"=w122:string)  [unwired: 13 in]
      }
      frame "Initialize Tasks" {
        n50 = call "Cont Acq Thermocouple Samples-Int Clk-Init.vi"("error in"=w143, "Rate"="Rate_T", "Physical Channel"="cDAQ1Mod1/ai0:15,cDAQ1Mod2/ai0:15,cDAQ1Mod3/ai0:15,cDAQ1Mod4/ai0:15,cDAQ1Mod5/ai0:15" ("name to assign")) -> ("error out"=w142:errorcluster, "Temp task out"=w134:refnum<k21>)  [unwired: 7 in]
        n51 = call "Cont Acq AI Samples-Int Clk-Init.vi"("error in"=w142, "Rate"="Rate_AI", "physical channels"="cDAQ1Mod6/ai0:5,cDAQ1Mod7/ai0:7,cDAQ1Mod7/ai16:23" ("name to assign")) -> ("error out"=w141:errorcluster, "AI task out"=w135:refnum<k21>)  [unwired: 7 in]
        n52 = Build Array(w134, w135) -> (w137:refnum<k21>[])
        n53 = Bundle By Name(cluster=w139, "Tasks In"=w137) -> (w138:T5)
        n54 = case shown="Error" w141 {
          tunnel: [_ " Macro: Exit" ("State(s) in Front (\"\")")] -> w140
          frame No Error {
          }
          frame Error {
          }
        }
        n55 = call <vilib>:"Add State(s) to Queue__jki_lib_state_machine.vi"("State(s) in Front (\"\")"=w140, "State(s) in (\"\")"=w145) -> ("States Out"=w144:string)  [unwired: 13 in]
      }
      frame "Data: Cleanup" {
        # "Cleanup any data and references, here.\n(this is called automatically, by the Macro: Exit)"
        n56 = Unbundle By Name(w151) -> ("Tasks In"=w148:refnum<k21>[])  [unwired: 1 out]
        n57 = for {
          tunnel: w150 -> [w159]
          tunnel: [w155] -> w149
          tunnel: w148 -> [w156] mode=indexing
          n58 = call <vilib>:"DAQmx Stop Task.vi"("task/channels in"=w156, "error in"=w159) -> ("task out"=w157:refnum<k21>, "error out"=w158:errorcluster)  [unwired: 12 in]
          n59 = call <vilib>:"DAQmx Clear Task.vi"("task in"=w157, "error in"=w158) -> ("error out"=w160:errorcluster)  [unwired: 13 in]
          n60 = call <vilib>:"Simple Error Handler.vi"("error in (no error)"=w160) -> ("error out"=w155:errorcluster)  [unwired: 4 in, 4 out]
        }
        n61 = control-ref of="Current VI Reference"() -> (w147:refnum<vi>)
        n62 = Close Reference(reference=w147, error in (no error)=w149) -> (error out=w152:errorcluster)
        n63 = call <vilib>:"Add State(s) to Queue__jki_lib_state_machine.vi"("State(s) in (\"\")"=w154) -> ("States Out"=w153:string)  [unwired: 14 in]
      }
      frame "---------- UI ----------" {
        # "Do not put any code in this frame.\n(It is a separator no-op. You can make a copy of this frame to create a new UI frame)"
        n64 = call <vilib>:"Add State(s) to Queue__jki_lib_state_machine.vi"("State(s) in (\"\")"=w164) -> ("States Out"=w163:string)  [unwired: 14 in]
      }
      frame "UI: Initialize" {
        w169 = T2 {"Mean"=99.0, " Std"=99.0, "Color Box"=16318226} ("Sensor")
        # "Initialize the User Interface, here.\n(this is called automatically, by the Macro: Init)"
        n65 = stacked-sequence {
          tunnel: "Panel 1" -> [w177]
          tunnel: w169 -> [w176]
          tunnel: [w175] -> w166
          tunnel: "Panel 2" -> [_]
          tunnel: "Panel 3" -> [_]
          tunnel: "Panel 4" -> [_]
          frame #0 {
            n66 = for {
              tunnel: w177 -> [w180] mode=indexing
              tunnel: w176 -> [w179]
              tunnel: [w178] -> w175 mode=indexing
              n67 = for {
                tunnel: w180 -> [w186] mode=indexing
                tunnel: w179 -> [w185]
                tunnel: [w181] -> w178 mode=indexing
                n68 = Unbundle(w185) -> ("Mean"=w184:dbl, "Std"=w183:dbl, "Color Box"=w182:u32)
                n69 = Bundle By Name(cluster=w186, "Mean"=w184, "Std"=w183, "Color Box"=w182) -> (w181:T2)
              }
            }
          }
        }
        n70 = local write "Panel 4"(w166) -> ()
        n71 = local write "Panel 1"(w166) -> ()
        n72 = local write "Panel 2"(w166) -> ()
        n73 = local write "Panel 3"(w166) -> ()
        n74 = call <vilib>:"Add State(s) to Queue__jki_lib_state_machine.vi"("State(s) in (\"\")"=w174) -> ("States Out"=w173:string)  [unwired: 14 in]
        "Gas Temp" <- w169
      }
      frame "UI: Cursor Set" {
        # "Argument"
        # "Set and Unset Cursor Busy.\n(Usage: \"UI: Cursor Set >> Busy|Idle\")"
        n75 = case shown="\"Idle\", Default" w187 {
          tunnel: w189 -> [w194 w196]
          tunnel: [w193 w195] -> w188
          frame "Idle", Default {
            n76 = call <vilib>:"Unset Busy.vi"("error in (no error)"=w194) -> ("error out"=w193:errorcluster)  [unwired: 10 in]
          }
          frame "Busy" {
            n77 = call <vilib>:"Set Busy.vi"("error in (no error)"=w196) -> ("error out"=w195:errorcluster)  [unwired: 9 in, 1 out]
          }
        }
        n78 = call <vilib>:"Add State(s) to Queue__jki_lib_state_machine.vi"("State(s) in (\"\")"=w192) -> ("States Out"=w191:string)  [unwired: 14 in]
      }
      frame "UI: Front Panel State" {
        # "Argument"
        # "Set Front Panel Open or Closed\n(Usage: \"UI: Front Panel State >> Open|Close\")"
        n79 = Unbundle By Name(w199) -> ("Core.Current VI Reference"=w198:refnum<vi>)
        n80 = case shown="\"Close\"" w197 {
          tunnel: w201 -> [w207 w220]
          tunnel: [w209 w221] -> w200
          tunnel: w198 -> [w208 w218]
          frame "Open", Default {
            n81 = property class="VI"(reference=w208, error in=w207) -> (reference out=w205:refnum<vi>, error out=w206:errorcluster, "Front Panel.Open"=w204:bool)
            n82 = case shown="False" w204 {
              tunnel: [w212 w215] -> w209
              tunnel: w206 -> [w211 w215]
              tunnel: w205 -> [w210 _]
              frame False {
                n83 = invoke class="VI" method="FP.Open"(reference=w210, error in=w211, "Activate"=TRUE, "State"=T4."Standard") -> (error out=w212:errorcluster)  [unwired: 1 in, 4 out]
              }
              frame True {
              }
            }
          }
          frame "Close" {
            n84 = property class="VI"(reference=w218, error in=w220) -> (reference out=w217:refnum<vi>, error out=w219:errorcluster, "Front Panel.Open"=w216:bool)
            n85 = case shown="True" w216 {
              tunnel: [w222 w225] -> w221
              tunnel: w219 -> [w222 w224]
              tunnel: w217 -> [_ w223]
              frame False {
              }
              frame True {
                n86 = invoke class="VI" method="FP.Close"(reference=w223, error in=w224) -> (error out=w225:errorcluster)  [unwired: 1 in, 2 out]
              }
            }
          }
        }
        n87 = call <vilib>:"Add State(s) to Queue__jki_lib_state_machine.vi"("State(s) in (\"\")"=w203) -> ("States Out"=w202:string)  [unwired: 14 in]
      }
      frame "---------- Macro ----------" {
        # "Do not put any code in this frame.\n(It is a separator no-op. You can make a copy of this frame to create a new Macro frame)"
        n88 = call <vilib>:"Add State(s) to Queue__jki_lib_state_machine.vi"("State(s) in (\"\")"=w229) -> ("States Out"=w228:string)  [unwired: 14 in]
      }
      frame "Macro: Initialize" {
        # "Initialization Macro\n(This is called once, when the VI starts)"
        n89 = call <vilib>:"Add State(s) to Queue__jki_lib_state_machine.vi"("State(s) in Front (\"\")"="Data: Initialize\nInitialize Tasks\nInitialize Core Data\nUI: Initialize\nUI: Front Panel State >> Open", "State(s) in (\"\")"=w234) -> ("States Out"=w233:string)  [unwired: 13 in]
      }
      frame "Macro: Exit" {
        # "Exit Macro\n(This is called once, when the VI exits)"
        n90 = Unbundle By Name(w241) -> ("Core.Close Panel on Exit?"=w240:bool)
        n91 = Select(t="UI: Front Panel State >> Close", s=w240, f="") -> (s? t:f=w237:string)
        n92 = call <vilib>:"Add State(s) to Queue__jki_lib_state_machine.vi"("State(s) in (\"\")"=w237, "State(s) at Back (\"\")"="Data: Cleanup\nExit") -> ("States Out"=w235:string)  [unwired: 13 in]
        n93 = call <vilib>:"Add State(s) to Queue__jki_lib_state_machine.vi"("State(s) in Front (\"\")"=w235, "State(s) in (\"\")"=w244) -> ("States Out"=w243:string)  [unwired: 13 in]
      }
      frame "---------- Main ----------" {
        # "Template Separator\n(You can make a copy of, or modify, this frame)"
        n94 = call <vilib>:"Add State(s) to Queue__jki_lib_state_machine.vi"("State(s) in (\"\")"=w248) -> ("States Out"=w247:string)  [unwired: 14 in]
      }
      frame "Test: TCs" {
        # "Your code here.\n(You can make a copy of, or modify, this frame)"
        n95 = call <vilib>:"Add State(s) to Queue__jki_lib_state_machine.vi"("State(s) in (\"\")"=w253, "State(s) at Back (\"\")"="TestDAQ: Gather Temps\nTestDAQ: Gather AI\nTestDAQ: Sort\nTestDAQ: Verify" ("State(s) at Back (\"\")")) -> ("States Out"=w252:string)  [unwired: 13 in]
      }
      frame "------ TestDAQ ------" {
        # "Template Separator\n(You can make a copy of, or modify, this frame)"
        n96 = call <vilib>:"Add State(s) to Queue__jki_lib_state_machine.vi"("State(s) in (\"\")"=w257) -> ("States Out"=w256:string)  [unwired: 14 in]
      }
      frame "TestDAQ: Gather Temps" {
        (unwired) -1 ("number of samples per channel")
        # "Template Separator\n(You can make a copy of, or modify, this frame)"
        n97 = Unbundle By Name(w273) -> ("Init"=w269:bool, "Tasks In"=w267:refnum<k21>[])
        n98 = Index Array(array=w267, index #1=0 ("index"), index #2=1 ("index")) -> (element #1=w263:refnum<k21>)  [unwired: 1 out]
        n99 = while {
          tunnel: w263 -> [w283]
          tunnel: [w281] -> w258
          tunnel: [w278] -> w259
          i -> [w276]
          stop <- w277 continue-if-true
          w280 = u32 5 ("y")
          n100 = property class="DAQmx Read"(reference=w283) -> (reference out=w278:refnum<k21>, "AvailSampPerChan"=w281:u32)  [unwired: 1 in, 1 out]
          n101 = Less?(x=w276, y=w280) -> (x < y?=w279:bool)
          n102 = Less?(x=w281, y=w280) -> (x < y?=w282:bool)
          n103 = And(x=w282, y=w279) -> (x .and. y?=w277:bool)
          n104 = case shown="True" w277 {
            frame False {
            }
            frame True {
              n105 = Wait (ms)(milliseconds to wait=u32 5) -> ()  [unwired: 1 out]
            }
          }
        }
        "AvailSampPerTempChan" <- w258
        n106 = call "Counter.vi"("Reset"=w269) -> ("Count"=→"Count":dbl)  [unwired: 10 in]
        n107 = call-poly <vilib>:"DAQmx Read.vi"("task/channels in"=w259, "number of samples per channel"=w258, "error in"=w260) -> ("data"=w262:dbl[][], "error out"=w261:errorcluster)  [unwired: 10 in, 1 out]
        "Temps data" <- w262
        n108 = case shown="Error" w261 {
          selector: w261 -> [_ w288]
          frame No Error {
          }
          frame Error {
            n109 = Unbundle(w288) -> ("source"=w286:string)  [unwired: 2 out]
            n110 = Concatenate Strings("temps:" ("message"), w286) -> (w285:string)
            n111 = Two Button Dialog(message=w285, 2:"exit" ("T button name (\"OK\")")) -> (T button?=w289:bool)  [unwired: 1 in]
            n112 = case shown="True" w289 {
              selector: w289 -> [_ w291]
              frame False {
              }
              frame True {
                n113 = Stop(stop? (T)=w291) -> ()
              }
            }
          }
        }
        n114 = for {
          tunnel: w262 -> [w296] mode=indexing
          tunnel: [w293] -> w272 mode=indexing
          tunnel: T2 {"Mean"=0.0, " Std"=0.0, "Color Box"=5373696} ("Sensor") -> [w292]
          n115 = call <vilib>:"Std Deviation and Variance.vi"("X"=w296) -> ("mean"=w295:dbl, "standard deviation"=w294:dbl)  [unwired: 1 in, 1 out]
          n116 = Bundle By Name(cluster=w292, "Mean"=w295, "Std"=w294) -> (w293:T2)
        }
        n117 = Bundle By Name(cluster=w273, "Init"=FALSE, "Temp  Data Array"=w272) -> (w271:T5)
        n118 = call <vilib>:"Add State(s) to Queue__jki_lib_state_machine.vi"("State(s) in (\"\")"=w275) -> ("States Out"=w274:string)  [unwired: 14 in]
      }
      frame "TestDAQ: Gather AI" {
        # "Template Separator\n(You can make a copy of, or modify, this frame)"
        n119 = Unbundle By Name(w315) -> ("Tasks In"=w311:refnum<k21>[])
        n120 = Index Array(array=w311, index #1=0 ("index"), index #2=1 ("index")) -> (element #2=w306:refnum<k21>)  [unwired: 1 out]
        n121 = while {
          tunnel: w306 -> [w325]
          tunnel: [w323] -> w304
          tunnel: [w320] -> w305
          i -> [w318]
          stop <- w319 continue-if-true
          w322 = u32 5 ("y")
          n122 = property class="DAQmx Read"(reference=w325) -> (reference out=w320:refnum<k21>, "AvailSampPerChan"=w323:u32)  [unwired: 1 in, 1 out]
          n123 = Less?(x=w318, y=w322) -> (x < y?=w321:bool)
          n124 = Less?(x=w323, y=w322) -> (x < y?=w324:bool)
          n125 = And(x=w324, y=w321) -> (x .and. y?=w319:bool)
          n126 = case shown="True" w319 {
            frame False {
            }
            frame True {
              n127 = Wait (ms)(milliseconds to wait=u32 5) -> ()  [unwired: 1 out]
            }
          }
        }
        "AvailSampPerAIChan" <- w304
        n128 = local read "I.DC Event"() -> (w301:i32)
        n129 = call-poly <vilib>:"DAQmx Read.vi"("task/channels in"=w305, "number of samples per channel"=w304, "error in"=w312) -> ("data"=w303:dbl[][], "error out"=w307:errorcluster)  [unwired: 10 in, 1 out]
        "AI Data" <- w303
        "Voltages" <- w303
        "error ai" <- w307
        n130 = Array Subset(array=w303, index (row)=w301, length (row)=8 ("length")) -> (w299:dbl[][])  [unwired: 2 in]
        n131 = call "File AI Stream Save.vi"("DC Voltages Filename"="DC Voltages Filename", "Array"=w299, "Enable"="Stream Voltages to File") -> ("new file path (Not A Path if cancelled)"=w297:path)  [unwired: 7 in, 1 out]
        n132 = local write "DC Voltages Filename"(w297) -> ()
        n133 = local read "G.Pres."() -> (w308:cluster{"Mean":dbl, "StdDev":dbl})
        n134 = for {
          tunnel: w303 -> [w331] mode=indexing
          tunnel: [w328] -> w314 mode=indexing
          tunnel: w308 -> [w327]
          n135 = call <vilib>:"Std Deviation and Variance.vi"("X"=w331) -> ("mean"=w330:dbl, "standard deviation"=w329:dbl)  [unwired: 1 in, 1 out]
          n136 = Bundle By Name(cluster=w327, "Mean"=w330, "StdDev"=w329) -> (w328:cluster{"Mean":dbl, "StdDev":dbl})
        }
        n137 = Bundle By Name(cluster=w315, "AI Data"=w314) -> (w313:T5)
        n138 = call <vilib>:"Add State(s) to Queue__jki_lib_state_machine.vi"("State(s) in (\"\")"=w317) -> ("States Out"=w316:string)  [unwired: 14 in]
      }
      frame "TestDAQ: Sort" {
        # "Analog Channels\nGs Pressure 0\nWeight 1\nRH 2\nGas Volume 3\nTemp 4\nBaromentric Pressure 5"
        # "Template Separator\n(You can make a copy of, or modify, this frame)"
        n139 = global read "Global Test Variables DPT.vi" "Globals for Dryer Performance Test"() -> (w353:T7)
        n140 = Unbundle By Name(w353) -> ("Test Setup.GPres4mA Val"=w340:dbl, "Test Setup.Gpres20mA Val"=w339:dbl, "Test Setup.Gas P. Resistor"=w338:dbl, "Test Setup.RH4mA Val"=w337:dbl, "Test Setup.RH20mA Val"=w336:dbl, "Test Setup.RH Resistor"=w335:dbl, "Test Setup.Temp4mA Val"=w334:dbl, "Test Setup.Temp20mA Val"=w333:dbl, "Test Setup.Temp Resistor"=w332:dbl, "cDAQ Array Locations.Gas Pressure"=w349:string, "cDAQ Array Locations.RH Chan"=w348:string, "cDAQ Array Locations.Temp Chan"=w347:string, "cDAQ Array Locations.Barometric Pressure"=w346:string, "cDAQ Array Locations.Gas Feedback Chan"=w345:string, "cDAQ Array Locations.Scale Channel"=w344:string, "cDAQ Array Locations.Gas Temperature"=w342:string, "cDAQ Array Locations.VDC Discrete Channel"=w341:string)  [unwired: 1 out]
        n141 = Unbundle By Name(w352) -> ("CDAQ Data"=w350:dbl[], "Temp  Data Array"=w355:T2[], "AI Data"=w354:cluster{"Mean":dbl, "StdDev":dbl}[])
        n142 = stacked-sequence {
          seq-local: [_ _ _ _ _ _ _ _ w516 _ _] -> [_ _ _ _ _ _ _ _ _ w584 _]
          seq-local: [_ _ _ _ _ _ _ _ _ w555 _] -> [_ _ _ _ _ _ _ _ _ _ w591]
          tunnel: w355 -> [w361 w382 w403 w422 w447 _ _ _ _ _ _]
          tunnel: w354 -> [_ _ _ _ _ w485 w508 w510 _ _ _]
          tunnel: w350 -> [_ _ _ _ _ _ _ _ w529 _ _]
          tunnel: w349 -> [_ _ _ _ _ _ _ _ _ w583 _]
          tunnel: w348 -> [_ _ _ _ _ _ _ _ _ w576 _]
          tunnel: w347 -> [_ _ _ _ _ _ _ _ _ w563 _]
          tunnel: w346 -> [_ _ _ _ _ _ _ _ _ w562 _]
          tunnel: w345 -> [_ _ _ _ _ _ _ _ _ w561 _]
          tunnel: w344 -> [_ _ _ _ _ _ _ _ _ w560 _]
          tunnel: [_ _ _ _ _ _ _ _ _ _ w592] -> w343
          tunnel: w342 -> [_ _ _ _ _ _ _ _ _ w557 _]
          tunnel: w341 -> [_ _ _ _ _ _ _ _ _ _ w589]
          tunnel: w340 -> [_ _ _ _ _ w460 _ _ _ _ _]
          tunnel: w339 -> [_ _ _ _ _ w459 _ _ _ _ _]
          tunnel: w338 -> [_ _ _ _ _ w458 _ _ _ _ _]
          tunnel: w337 -> [_ _ _ _ _ w457 _ _ _ _ _]
          tunnel: w336 -> [_ _ _ _ _ w456 _ _ _ _ _]
          tunnel: w335 -> [_ _ _ _ _ w455 _ _ _ _ _]
          tunnel: w334 -> [_ _ _ _ _ w454 _ _ _ _ _]
          tunnel: w333 -> [_ _ _ _ _ w453 _ _ _ _ _]
          tunnel: w332 -> [_ _ _ _ _ w452 _ _ _ _ _]
          frame #0 {
            n143 = local read "Panel 1"() -> (w366:T2[][])
            n144 = Array Subset(array=w361, index=1, length=6) -> (w368:T2[])
            n145 = Array Subset(array=w361, index=64, length=3) -> (w359:T2[])
            n146 = Array Subset(array=w361, index=7, length=6) -> (w365:T2[])
            n147 = Array Subset(array=w361, index=13, length=3) -> (w364:T2[])
            n148 = Replace Array Subset(array=w366, new element=w368, index (row)=0) -> (w377:T2[][])  [unwired: 1 in]
            n149 = Build Array (concatenate)(w364, w359) -> (w360:T2[])
            n150 = Replace Array Subset(array=w377, new element=w365, index (row)=1) -> (w375:T2[][])  [unwired: 1 in]
            n151 = Replace Array Subset(array=w375, new element=w360, index (row)=2) -> (w367:T2[][])  [unwired: 1 in]
            n152 = local write "Panel 1"(w367) -> ()
          }
          frame #1 {
            n153 = local read "Panel 2"() -> (w386:T2[][])
            n154 = Array Subset(array=w382, index=16, length=6) -> (w389:T2[])
            n155 = Array Subset(array=w382, index=22, length=6) -> (w388:T2[])
            n156 = Array Subset(array=w382, index=28, length=4) -> (w387:T2[])
            n157 = Array Subset(array=w382, index=67, length=2) -> (w380:T2[])
            n158 = Replace Array Subset(array=w386, new element=w389, index (row)=0) -> (w398:T2[][])  [unwired: 1 in]
            n159 = Build Array (concatenate)(w387, w380) -> (w381:T2[])
            n160 = Replace Array Subset(array=w398, new element=w388, index (row)=1) -> (w396:T2[][])  [unwired: 1 in]
            n161 = Replace Array Subset(array=w396, new element=w381, index (row)=2) -> (w385:T2[][])  [unwired: 1 in]
            n162 = local write "Panel 2"(w385) -> ()
          }
          frame #2 {
            n163 = local read "Panel 3"() -> (w407:T2[][])
            n164 = Array Subset(array=w403, index=69, length=2) -> (w401:T2[])
            n165 = Array Subset(array=w403, index=32, length=6) -> (w410:T2[])
            n166 = Array Subset(array=w403, index=38, length=6) -> (w409:T2[])
            n167 = Array Subset(array=w403, index=44, length=4) -> (w408:T2[])
            n168 = Replace Array Subset(array=w407, new element=w410, index (row)=0) -> (w419:T2[][])  [unwired: 1 in]
            n169 = Build Array (concatenate)(w408, w401) -> (w402:T2[])
            n170 = Replace Array Subset(array=w419, new element=w409, index (row)=1) -> (w417:T2[][])  [unwired: 1 in]
            n171 = Replace Array Subset(array=w417, new element=w402, index (row)=2) -> (w406:T2[][])  [unwired: 1 in]
            n172 = local write "Panel 3"(w406) -> ()
          }
          frame #3 {
            n173 = local read "Panel 4"() -> (w429:T2[][])
            n174 = Array Subset(array=w422, index=48, length=6) -> (w431:T2[])
            n175 = Array Subset(array=w422, index=54, length=6) -> (w430:T2[])
            n176 = Array Subset(array=w422, index=60, length=4) -> (w425:T2[])
            n177 = Array Subset(array=w422, index=71, length=2) -> (w423:T2[])
            n178 = Replace Array Subset(array=w429, new element=w431, index (row)=0) -> (w440:T2[][])  [unwired: 1 in]
            n179 = Build Array (concatenate)(w425, w423) -> (w424:T2[])
            n180 = Replace Array Subset(array=w440, new element=w430, index (row)=1) -> (w438:T2[][])  [unwired: 1 in]
            n181 = Replace Array Subset(array=w438, new element=w424, index (row)=2) -> (w428:T2[][])  [unwired: 1 in]
            n182 = local write "Panel 4"(w428) -> ()
          }
          frame #4 {
            n183 = Index Array(array=w447, index #1=35 ("index"), index #2=33 ("index"), index #3=34 ("length")) -> ()  [unwired: 3 out]
            n184 = Array Subset(array=w447, index=17, length=3) -> ()  [unwired: 1 out]
            n185 = Index Array(array=w447, index=0) -> (element=w446:T2)
            n186 = Index Array(array=w447, index=15) -> ()  [unwired: 1 out]
            n187 = local write "Gas Temp"(w446) -> ()
          }
          frame #5 {
            n188 = call "Scale 4-20 sig.vi"("4 mA value"=w460, "20 mA value"=w459, "Drop resistor"=w458) -> ("M"=w483:dbl, "B"=w472:dbl)  [unwired: 11 in]
            n189 = call "Scale 4-20 sig.vi"("4 mA value"=w457, "20 mA value"=w456, "Drop resistor"=w455) -> ("M"=w479:dbl, "B"=w468:dbl)  [unwired: 11 in]
            n190 = call "Scale 4-20 sig.vi"("4 mA value"=w454, "20 mA value"=w453, "Drop resistor"=w452) -> ("M"=w475:dbl, "B"=w462:dbl)  [unwired: 11 in]
            n191 = Index Array(array=w485, index #1="I.Gas Pressure", index #2="I.RH", index #3="I.Tmp") -> (element #1=w482:cluster{"Mean":dbl, "StdDev":dbl}, element #2=w478:cluster{"Mean":dbl, "StdDev":dbl}, element #3=w473:cluster{"Mean":dbl, "StdDev":dbl})
            n192 = Multiply(x=w478, y=w479) -> (x*y=w466:cluster{"Mean":dbl, "StdDev":dbl})
            n193 = Multiply(x=w473, y=w475) -> (x*y=w463:cluster{"Mean":dbl, "StdDev":dbl})
            n194 = Multiply(x=w482, y=w483) -> (x*y=w471:cluster{"Mean":dbl, "StdDev":dbl})
            n195 = Bundle(cluster=w466, "Mean"=w468, "StdDev"=0.0) -> (w467:cluster{"Mean":dbl, "StdDev":dbl})
            n196 = Bundle(cluster=w471, "Mean"=w472, "StdDev"=0.0) -> (w470:cluster{"Mean":dbl, "StdDev":dbl})
            n197 = Bundle(cluster=w463, "Mean"=w462, "StdDev"=0.0) -> (w464:cluster{"Mean":dbl, "StdDev":dbl})
            n198 = Add(x=w471, y=w470) -> (x+y=→"G.Pres.":cluster{"Mean":dbl, "StdDev":dbl})
            n199 = Add(x=w466, y=w467) -> (x+y=→"RH":cluster{"Mean":dbl, "StdDev":dbl})
            n200 = Add(x=w463, y=w464) -> (x+y=→"Temp":cluster{"Mean":dbl, "StdDev":dbl})
          }
          frame #6 {
            w498 = 3.0  # Gas Volume Scale
            # "30 ft3 = 10v"
            n201 = Index Array(array=w508, index #1="I.Bar", index #2="I.Gvol", index #3="I.W") -> (element #1=w506:cluster{"Mean":dbl, "StdDev":dbl}, element #2=w503:cluster{"Mean":dbl, "StdDev":dbl}, element #3=w500:cluster{"Mean":dbl, "StdDev":dbl})
            n202 = Multiply(x=w506, y=1.5 ("4 mA value")) -> (x*y=w496:cluster{"Mean":dbl, "StdDev":dbl})
            n203 = Multiply(x=w503, y=w498) -> (x*y=w504:cluster{"Mean":dbl, "StdDev":dbl})
            n204 = Multiply(x=w500, y=15.0 ("4 mA value")) -> (x*y=w486:cluster{"Mean":dbl, "StdDev":dbl})
            n205 = Add(x=w504, y=0.0 ("4 mA value")) -> (x+y=w491:cluster{"Mean":dbl, "StdDev":dbl})
            "G.Vol" <- w491
            n206 = Bundle(cluster=w496, "Mean"=20.0 ("4 mA value"), "StdDev"=0.0) -> (w493:cluster{"Mean":dbl, "StdDev":dbl})
            n207 = Bundle(cluster=w491, "Mean"=50.0 ("4 mA value"), "StdDev"=0.0) -> (w488:cluster{"Mean":dbl, "StdDev":dbl})
            n208 = Add(x=w496, y=w493) -> (x+y=→"Bar":cluster{"Mean":dbl, "StdDev":dbl})
            n209 = Add(x=w486, y=w488) -> (x+y=→"Weight":cluster{"Mean":dbl, "StdDev":dbl})
          }
          frame #7 {
            w511 = 8 ("length")
            n210 = Delete From Array(array=w510, length=w511, index="I.AC Event") -> (deleted portion=→"AC Events":cluster{"Mean":dbl, "StdDev":dbl}[])  [unwired: 1 out]
            n211 = Delete From Array(array=w510, length=w511, index="I.DC Event") -> (deleted portion=→"DC Voltages":cluster{"Mean":dbl, "StdDev":dbl}[])  [unwired: 1 out]
          }
          frame #8 {
            n212 = local read "Panel 1"() -> (w530:T2[][])
            n213 = local read "Panel 2"() -> (w526:T2[][])
            n214 = local read "Panel 3"() -> (w524:T2[][])
            n215 = local read "Panel 4"() -> (w522:T2[][])
            n216 = for {
              tunnel: w530 -> [w552] mode=indexing
              shift-right: [w550] -> w518
              shift-left: dbl[] [] -> [w549]
              n217 = for {
                tunnel: w552 -> [w554] mode=indexing
                tunnel: [w553] -> w551 mode=indexing
                n218 = Unbundle By Name(w554) -> ("Mean"=w553:dbl)
              }
              n219 = Build Array (concatenate)(w549, w551) -> (w550:dbl[])
            }
            n220 = for {
              tunnel: w526 -> [w546] mode=indexing
              shift-right: [w544] -> w521
              shift-left: dbl[] [] -> [w543]
              n221 = for {
                tunnel: w546 -> [w548] mode=indexing
                tunnel: [w547] -> w545 mode=indexing
                n222 = Unbundle By Name(w548) -> ("Mean"=w547:dbl)
              }
              n223 = Build Array (concatenate)(w543, w545) -> (w544:dbl[])
            }
            n224 = for {
              tunnel: w524 -> [w540] mode=indexing
              shift-right: [w538] -> w520
              shift-left: dbl[] [] -> [w537]
              n225 = for {
                tunnel: w540 -> [w542] mode=indexing
                tunnel: [w541] -> w539 mode=indexing
                n226 = Unbundle By Name(w542) -> ("Mean"=w541:dbl)
              }
              n227 = Build Array (concatenate)(w537, w539) -> (w538:dbl[])
            }
            n228 = for {
              tunnel: w522 -> [w534] mode=indexing
              shift-right: [w532] -> w519
              shift-left: dbl[] [] -> [w531]
              n229 = for {
                tunnel: w534 -> [w536] mode=indexing
                tunnel: [w535] -> w533 mode=indexing
                n230 = Unbundle By Name(w536) -> ("Mean"=w535:dbl)
              }
              n231 = Build Array (concatenate)(w531, w533) -> (w532:dbl[])
            }
            n232 = Build Array (concatenate)(w518, w521, w520, w519) -> (w517:dbl[])
            n233 = Replace Array Subset(array=w529, new element=w517, index=0) -> (w516:dbl[])
          }
          frame #9 {
            n234 = local read "Gas Temp"() -> (w559:T2)
            n235 = local read "G.Pres."() -> (w581:cluster{"Mean":dbl, "StdDev":dbl})
            n236 = local read "Weight"() -> (w564:cluster{"Mean":dbl, "StdDev":dbl})
            n237 = local read "Temp"() -> (w567:cluster{"Mean":dbl, "StdDev":dbl})
            n238 = local read "G.Vol"() -> (w565:cluster{"Mean":dbl, "StdDev":dbl})
            n239 = local read "Bar"() -> (w566:cluster{"Mean":dbl, "StdDev":dbl})
            n240 = local read "RH"() -> (w577:cluster{"Mean":dbl, "StdDev":dbl})
            n241 = Unbundle By Name(w577) -> ("Mean"=w579:dbl)
            n242 = Unbundle By Name(w581) -> ("Mean"=w580:dbl)
            n243 = Unbundle By Name(w565) -> ("Mean"=w574:dbl)
            n244 = Unbundle By Name(w567) -> ("Mean"=w572:dbl)
            n245 = Unbundle By Name(w566) -> ("Mean"=w573:dbl)
            n246 = Decimal String To Number(string=w583) -> (number=w582:i32)  [unwired: 2 in, 1 out]
            n247 = Unbundle By Name(w564) -> ("Mean"=w575:dbl)
            n248 = Decimal String To Number(string=w576) -> (number=w578:i32)  [unwired: 2 in, 1 out]
            n249 = Decimal String To Number(string=w561) -> (number=w569:i32)  [unwired: 2 in, 1 out]
            n250 = Decimal String To Number(string=w563) -> (number=w571:i32)  [unwired: 2 in, 1 out]
            n251 = Decimal String To Number(string=w562) -> (number=w570:i32)  [unwired: 2 in, 1 out]
            n252 = Decimal String To Number(string=w560) -> (number=w568:i32)  [unwired: 2 in, 1 out]
            n253 = Decimal String To Number(string=w557) -> (number=w556:i32)  [unwired: 2 in, 1 out]
            n254 = Unbundle By Name(w559) -> ("Mean"=w558:dbl)
            n255 = Replace Array Subset(array=w584, new element #1=w580, index #1=w582, new element #2=w579, index #2=w578, new element #3=w572, index #3=w571, new element #4=w573, index #4=w570, new element #5=w574, index #5=w569, new element #6=w575, index #6=w568, new element #7=w558, index #7=w556) -> (w555:dbl[])
          }
          frame #10 {
            n256 = local read "DC Voltages"() -> (w588:cluster{"Mean":dbl, "StdDev":dbl}[])
            n257 = local read "AC Events"() -> (w587:cluster{"Mean":dbl, "StdDev":dbl}[])
            n258 = Build Array (concatenate)(w588, w587) -> (w586:cluster{"Mean":dbl, "StdDev":dbl}[])
            n259 = for {
              tunnel: w586 -> [w594] mode=indexing
              tunnel: [w593] -> w585 mode=indexing
              n260 = Unbundle By Name(w594) -> ("Mean"=w593:dbl)
            }
            n261 = Decimal String To Number(string=w589) -> (number=w590:i32)  [unwired: 2 in, 1 out]
            n262 = Replace Array Subset(array=w591, new element=w585, index=w590) -> (w592:dbl[])
          }
        }
        n263 = Bundle By Name(cluster=w352, "CDAQ Data"=w343) -> (w351:T5)
        n264 = local write "CDAQ Data Out"(w343) -> ()
        n265 = call <vilib>:"Add State(s) to Queue__jki_lib_state_machine.vi"("State(s) in (\"\")"=w358) -> ("States Out"=w357:string)  [unwired: 14 in]
      }
      frame "TestDAQ: Verify" {
        # "Template Separator\n(You can make a copy of, or modify, this frame)"
        n266 = local read "Panel 4"() -> (w598:T2[][])
        n267 = local read "Panel 3"() -> (w599:T2[][])
        n268 = local read "Panel 1"() -> (w601:T2[][])
        n269 = local read "Panel 2"() -> (w600:T2[][])
        n270 = stacked-sequence {
          tunnel: w600 -> [_ w615 _ _]
          tunnel: w601 -> [w609 _ _ _]
          tunnel: w599 -> [_ _ w620 _]
          tunnel: w598 -> [_ _ _ w625]
          tunnel: "TC Min OK Val" -> [w608 w611 w616 w621]
          tunnel: "TC Max OK Val" -> [w607 w612 w617 w622]
          tunnel: "StDev Thresh" -> [w606 w613 w618 w623]
          frame #0 {
            n271 = call "Panel Color Set.vi"("TC Min OK Val"=w608, "TC Max OK Val"=w607, "StDev Thresh"=w606, "Panel 1"=w609) -> ("Panel Out"=w610:T2[][])
            n272 = local write "Panel 1"(w610) -> ()
          }
          frame #1 {
            n273 = call "Panel Color Set.vi"("TC Min OK Val"=w611, "TC Max OK Val"=w612, "StDev Thresh"=w613, "Panel 1"=w615) -> ("Panel Out"=w614:T2[][])
            n274 = local write "Panel 2"(w614) -> ()
          }
          frame #2 {
            n275 = call "Panel Color Set.vi"("TC Min OK Val"=w616, "TC Max OK Val"=w617, "StDev Thresh"=w618, "Panel 1"=w620) -> ("Panel Out"=w619:T2[][])
            n276 = local write "Panel 3"(w619) -> ()
          }
          frame #3 {
            n277 = call "Panel Color Set.vi"("TC Min OK Val"=w621, "TC Max OK Val"=w622, "StDev Thresh"=w623, "Panel 1"=w625) -> ("Panel Out"=w624:T2[][])
            n278 = local write "Panel 4"(w624) -> ()
          }
        }
        n279 = call <vilib>:"Add State(s) to Queue__jki_lib_state_machine.vi"("State(s) in (\"\")"=w605) -> ("States Out"=w604:string)  [unwired: 14 in]
      }
    }
  }
  n280 = disable-structure shown="Enabled" {
    disable-tunnel: w3 -> [w626 _]
    frame Disabled {
      n281 = case shown="\"Exe\"" w626 {
        frame "Exe" {
          n282 = while {
            stop <- "End" stop-if-true
            n283 = event shown="[0] Timeout" {
              selector: _ -> [_]
              dyn-events: _ -> [_]
              timeout: 150 -> [_]
              event Timeout {
                n284 = event-data() -> ()  [unwired: 1 in, 2 out]
              }
            }
          }
        }
        frame "Init CDAQ", Default {
        }
      }
    }
    frame Enabled {
    }
  }
  n285 = Unbundle By Name(w5) -> ("CDAQ Data"=→"CDAQ Data Out":dbl[], "Tasks In"=w2:refnum<k21>[], "error in (no error)"=→"error out":errorcluster)
  "Tasks Out" <- w2
  n286 = local write "Tasks In"(w2) -> ()
